vi "0 OCU.vi"(9 "Overview Image Ref In":T11, 10 "Map Name":T3="LPB Pool", 11 "Location of THINK":T14="127.0.0.1") -> ()   [LabVIEW 2011]
doc: "This is the current implementation of the operator control unit (OCU) for sailbot interfacing with this OCU over a network connection. The following features are currently implemented:\n- override control of the rudden angle and sail value by control interface or using keys\n- ability to add missions before and during a run, by clicking and by using GPS location of the boat or an auxiliary GPS attached to the OCU computer\n- modification of tuning values used on the boat\n- indicators for all relevant system status information\n\nAuthors: Jared Kirschner, Jason Curtis"
uses:
  2-Think/2 Typedefs/setpoints to boat.ctl
  2-Think/2 Typedefs/sail setpt.ctl
  2-Think/2 Typedefs/rudder angle.ctl
  2-Think/2 Typedefs/Velocity.ctl
  2-Think/2 Typedefs/apparent wind direction.ctl
  2-Think/2 Typedefs/apparent wind speed.ctl
  2-Think/2 Typedefs/apparent wind.ctl
  2-Think/2 Typedefs/heading.ctl
  2-Think/2 Typedefs/UTM Location.ctl
  2-Think/2 Typedefs/Which Boat.ctl
  2-Think/2 Typedefs/generalized sensor status.ctl
  2-Think/2 Typedefs/indicator LED.ctl
  0x2-OCU-Think Comm/0x2 Typedefs/Current Waypoint.ctl
  2-Think/2 Typedefs/robot velocity.ctl
  0x2-OCU-Think Comm/0x2 Typedefs/manual override.ctl
  0 Typedefs/Location of Think.ctl
  0 Typedefs/Sail Position.ctl
  0 Typedefs/Rudder Position.ctl
  0 Typedefs/Apparent Wind Point of Sail.ctl
  0x2-OCU-Think Comm/0x2 Typedefs/ocuWaypoint.ctl
  0x2-OCU-Think Comm/0x2 Typedefs/Waypoints List.ctl
  2-Think/2 Classes/Waypoint/Waypoint.lvclass
  0 Typedefs/Mission Type Radio Buttons.ctl
  2-Think/2 Typedefs/rate of turn.ctl
  2-Think/2 Typedefs/pitch and roll.ctl
  0 Typedefs/Maps.ctl
  <vilib>/vision/Image Controls.llb/IMAQ Image.ctl
  2-Think/2 Classes/Missions/GenericMission/GenericMission.lvclass
  2-Think/2 Typedefs/UTM Circle.ctl
  0x2-OCU-Think Comm/0x2 Typedefs/Control values.ctl
  2-Think/2 Typedefs/Goodness Weightings.ctl
  2-Think/2 Typedefs/PI Constants.ctl
  2-Think/2 Typedefs/Apparent Wind Mode.ctl
  0x2-OCU-Think Comm/0x2 Typedefs/Sail Setting Tuning.ctl
  2-Think/2 Typedefs/eStopCommand.ctl
  0x2-OCU-Think Comm/0x2 Typedefs/RIO-OCU update controls.ctl
  2-Think/2 Typedefs/generalized actuator status.ctl
  2-Think/2 Typedefs/absolute wind direction.ctl
  2-Think/2 Typedefs/absolute wind speed.ctl
  2-Think/2 Typedefs/absolute water current vector.ctl
  2-Think/2 Typedefs/Goodness Fns Indicator.ctl
  2-Think/2 Typedefs/tacking attempt.ctl
  0x2-OCU-Think Comm/0x2 Classes/NetworkStreams/Reader/readType.ctl
  0x2-OCU-Think Comm/0x2 Typedefs/ocuMessage.ctl
  0x2-OCU-Think Comm/0x2 Typedefs/ocuCommands.ctl
  2-Think/2 Globals/2 Global.vi
  0x2-OCU-Think Comm/OCUtoSim.vi
  0x2-OCU-Think Comm/0x2 Classes/NetworkStreams/Reader/NetworkStreamReader.lvclass
  0x2-OCU-Think Comm/0x2 Classes/NetworkStreams/Writer/NetworkStreamWriter.lvclass
  2-Think/2 Classes/Missions/RoundBuoy/RoundBuoy.lvclass
  2-Think/2 Classes/Missions/PassBuoys/PassBuoys.lvclass
  2-Think/2 Classes/Missions/StationKeeping/StationKeeping.lvclass
  2-Think/2 Classes/Missions/Drive/DriveTo.lvclass
panel:
  in  "Simulator controls":enum32{"Running", "Paused"}(tab)
  in  "Set Water Current Speed":dbl
  in  "Set Water Current Direction":dbl(knob) scale=0.0..360.0
  in  "Set Wind Speed":dbl=2.0
  in  "Pause Simulator?":bool
  in  "Set Wind Direction":dbl(knob) scale=0.0..360.0
  in  "Move boat?":bool
  in  "Set Boat Heading":dbl(knob) scale=0.0..360.0
  in  "Enable \nLocal GPS":bool
  out "Sensor Status":T1
  in  "GPS COM port":refnum<visa-resource-name>="COM1"
  in  "Additional inputs":T4(tab)
  in  "Manual Mission Input":enum32{"Drive", "Round", "Pass", "Station"}(tab)
  in  "Waypoint Location":enum32{"0", "1", "2", "3", "4"}(radio)
  in  "Buoy Side":enum32{"Starboard", "Port"}(radio)
  in  "Buoy to Round":enum32{"0", "1", "2", "3", "4"}(radio)
  in  "Starboard Buoy":enum32{"0", "1", "2", "3", "4"}(radio)=enum."1"
  in  "Port Buoy":enum32{"0", "1", "2", "3", "4"}(radio)
  in  "Buoy B":enum32{"0", "1", "2", "3", "4"}(radio)=enum."1"
  in  "Buoy A":enum32{"0", "1", "2", "3", "4"}(radio)
  in  "Add Mission":bool
  in  "Stored Locations Array":T5[](array[typedef])=[{"UTM Zone"=0.0, "Hemisphere"=enum."North", "East"=0.0, "North"=0.0}, {"UTM Zone"=0.0, "Hemisphere"=enum."North", "East"=0.0, "North"=0.0}, {"UTM Zone"=0.0, "Hemisphere"=enum."North", "East"=0.0, "North"=0.0}, {"UTM Zone"=0.0, "Hemisphere"=enum."North", "East"=0.0, "North"=0.0}, {"UTM Zone"=0.0, "Hemisphere"=enum."North", "East"=0.0, "North"=0.0}] {"North" format="%#_10f"; "East" format="%#_8f"}
  in  "Boat to Point 0":bool
  in  "Boat to Point 1":bool
  in  "Boat to Point 2":bool
  in  "Boat to Point 3":bool
  in  "Boat to Point 4":bool
  in  "Local to Point 4":bool
  in  "Local to Point 3":bool
  in  "Local to Point 2":bool
  in  "Local to Point 1":bool
  in  "Local to Point 0":bool
  in  "Update Constants":bool
  in  "Tuning Values":T6={"Goodness Weightings"={"Target Importance"=0.8, "No Sail Importance"=1.0, "Change Importance"=0.8, "Pure Waypoint \nImportance"=0.0, "Pure Wind \nImportance"=0.0}, "PI Constants"={"Proportional Gain"=0.5, "Integral Time"=0.0, "Derivative Time"=0.0}, "No Sail Zone\nTuning Quotient"=0.05, "Heading Change Wind Adjustment"=0.2, "Waypoint Tuning Quotient"=10.0, "Apparent Wind Mode"={"Desired Apparent\nWind Direction"=0.0, "On"=FALSE}, "Let Sail Out on Windcross"=TRUE, "Shift Goal for currents"=FALSE, "Round Buoy Safety"=5.0, "Sail Setting Options"={"Linear\nMode"=FALSE, "Sails Full In Point"=85.0, "Sails Full Out Point"=180.0}, "Defilter Wind Data"=TRUE, "Irons Range"=10.0, "Aggressiveness"=0.0} {"Aggressiveness" min=0.0 max=1.0; "Sail Setting Options"."Sails Full Out Point" step=0.1; "Sail Setting Options"."Sails Full In Point" step=0.1; "Apparent Wind Mode"."Desired Apparent\nWind Direction" step=0.1; "Goodness Weightings"."Pure Wind \nImportance" min=0.0 step=0.2; "Goodness Weightings"."Pure Waypoint \nImportance" min=0.0 step=0.2; "Goodness Weightings"."Change Importance" min=0.0 step=0.2; "Goodness Weightings"."No Sail Importance" min=0.0 step=0.2; "Goodness Weightings"."Target Importance" min=0.0 step=0.2}
  out "Battery Voltage":dbl
  out "Which Boat Am I?":T12
  out "Rudder Position":T13 scale=50.0..-50.0 scale format="%#.2g"
  out "Connected?":bool caption="Connection Status"
  in  "OVERRIDE SAIL?":bool
  in  "OVERRIDE RUDDER?":bool
  in  "Stop":bool
  in  "OCU Tab Control":enum32{"Mission [M]ap", "Detailed [T]elemetry"}(tab)
  in  "Map Mode":enum32{"M[i]ssion Edit", "M[o]nitoring"}(tab)
  in  "Load MDF":bool
  in  "Time(s)":dbl=300.0
  in  "Tolerance":dbl=3.0
  in  "Mission Entry Type":T15
  in  "Mission Def Filepath":path caption="MDF (Mission Definition File) path"
  in  "Reset Missions/Waypts":bool
  in  "Save Waypoints\nand PoI":bool
  out "Heading":T16 format="%05.1f"
  in  "Plot Colors":T17={"Target"=3381759, "No Sail"=16711680, "Change"=16756736, "Pure Waypt"=35080, "Pure Wind"=16860, "Combined"=16777228}
  out "Goodness Functions":picture
  out "Apparent Wind Direction\nPoint of Sail":T18 scale=0.0..360.0 scale format="%4d"
  out "Mission Status":string caption="Current Mission\nStatus"
  in  "Log message":string caption="Log message (type and press enter)"
  in  "Save Image":bool
  out "Mission Map":T11(plugin-control)
  in  "Overlay Font Size":i16=40
  out "# of Waypts":i32
  in  "Globals":T19(tab)
  out "Don't Tip?":bool
  out "Wind Sensor Status":T1
  out "Estimated Error":dbl
  out "Robot Heading":T16 format="%05.1f"
  out "Robot UTM Location":T5 {"North" format="%#_10f"; "East" format="%#_8f"}
  out "Robot Velocity":T20
  out "Robot\nRate of Turn":T21 format="%05.1f"
  out "Robot Pitch/Roll":T22 {"Roll" format="%05.1f"; "Pitch" format="%05.1f"}
  out "Robot Speed (m/s)":dbl
  out "Absolute Wind":T23 {"East" format="%#_5g"}
  out "Apparent Wind Direction":T24
  out "Apparent Wind Speed":T25
  out "Apparent Wind":T26
  out "Crossing Wind":bool
  out "Setpoints to boat":T27
  out "Sail Position":T28
  out "Rudder Angle":T29
  out "Current Waypoint":T30
  in  "Reset to start":bool
  out "Manual Override":T31
  out "Waypoints Array":T32[](array[typedef]) {"UTM Location"."North" format="%#_10f"; "UTM Location"."East" format="%#_8f"}
  out "Waypoints Object Array":T33
  out "Mission Object Array":refnum<class "GenericMission.lvclass">[](array[class])
  out "Global No Sail Circles":T34[](array[typedef])
  out "Sail Position":T35
  # "PORT"
  # "STARB"
  # "Local GPS"
  # "Note: if THINK\nis on this computer,\nturning on local GPS will do strange things."
  # "Note: the direction the current is coming from is opposite\n the dial. This is the direction the current is going to."
  # "When set,\nclick on map\nto move boat"
  # "HOWTO:\n1. save one or more points by moving GPS sensor to point, and pressing buttons below\n2. choose type of mission from tab control\n3. choose saved point(s) to load into mission. other params come from mission map input above\n4. click \"Add Mission\""
  # "P"
  # "S"
  # "O"
  # "O"
  # "A"
  # "B"
  # "HOWTO:\nchange values here, \nthen hit:"
  # "inputting missions:\nGo To Waypoint: set tolerance, and click on map.\nRound Buoy Port/Starboard: set tolerance, click.\nPass Between Buoys: Click one buoy location\nand drag to the other.\nStation Keeping: click southwest corner, drag to \nsoutheast corner. A square will be generated.\nTime(s) currently unimplemented.\nGlobal No-Sail Zone: click center of zone, drag to edge of\nzone. A circle with appropriate radius will be created."
  # "As Measured"
  # "Path Planning"
  # "From Planning Functions"
  # "(this is not a cluster because subitems\nare generated in parallel code)"
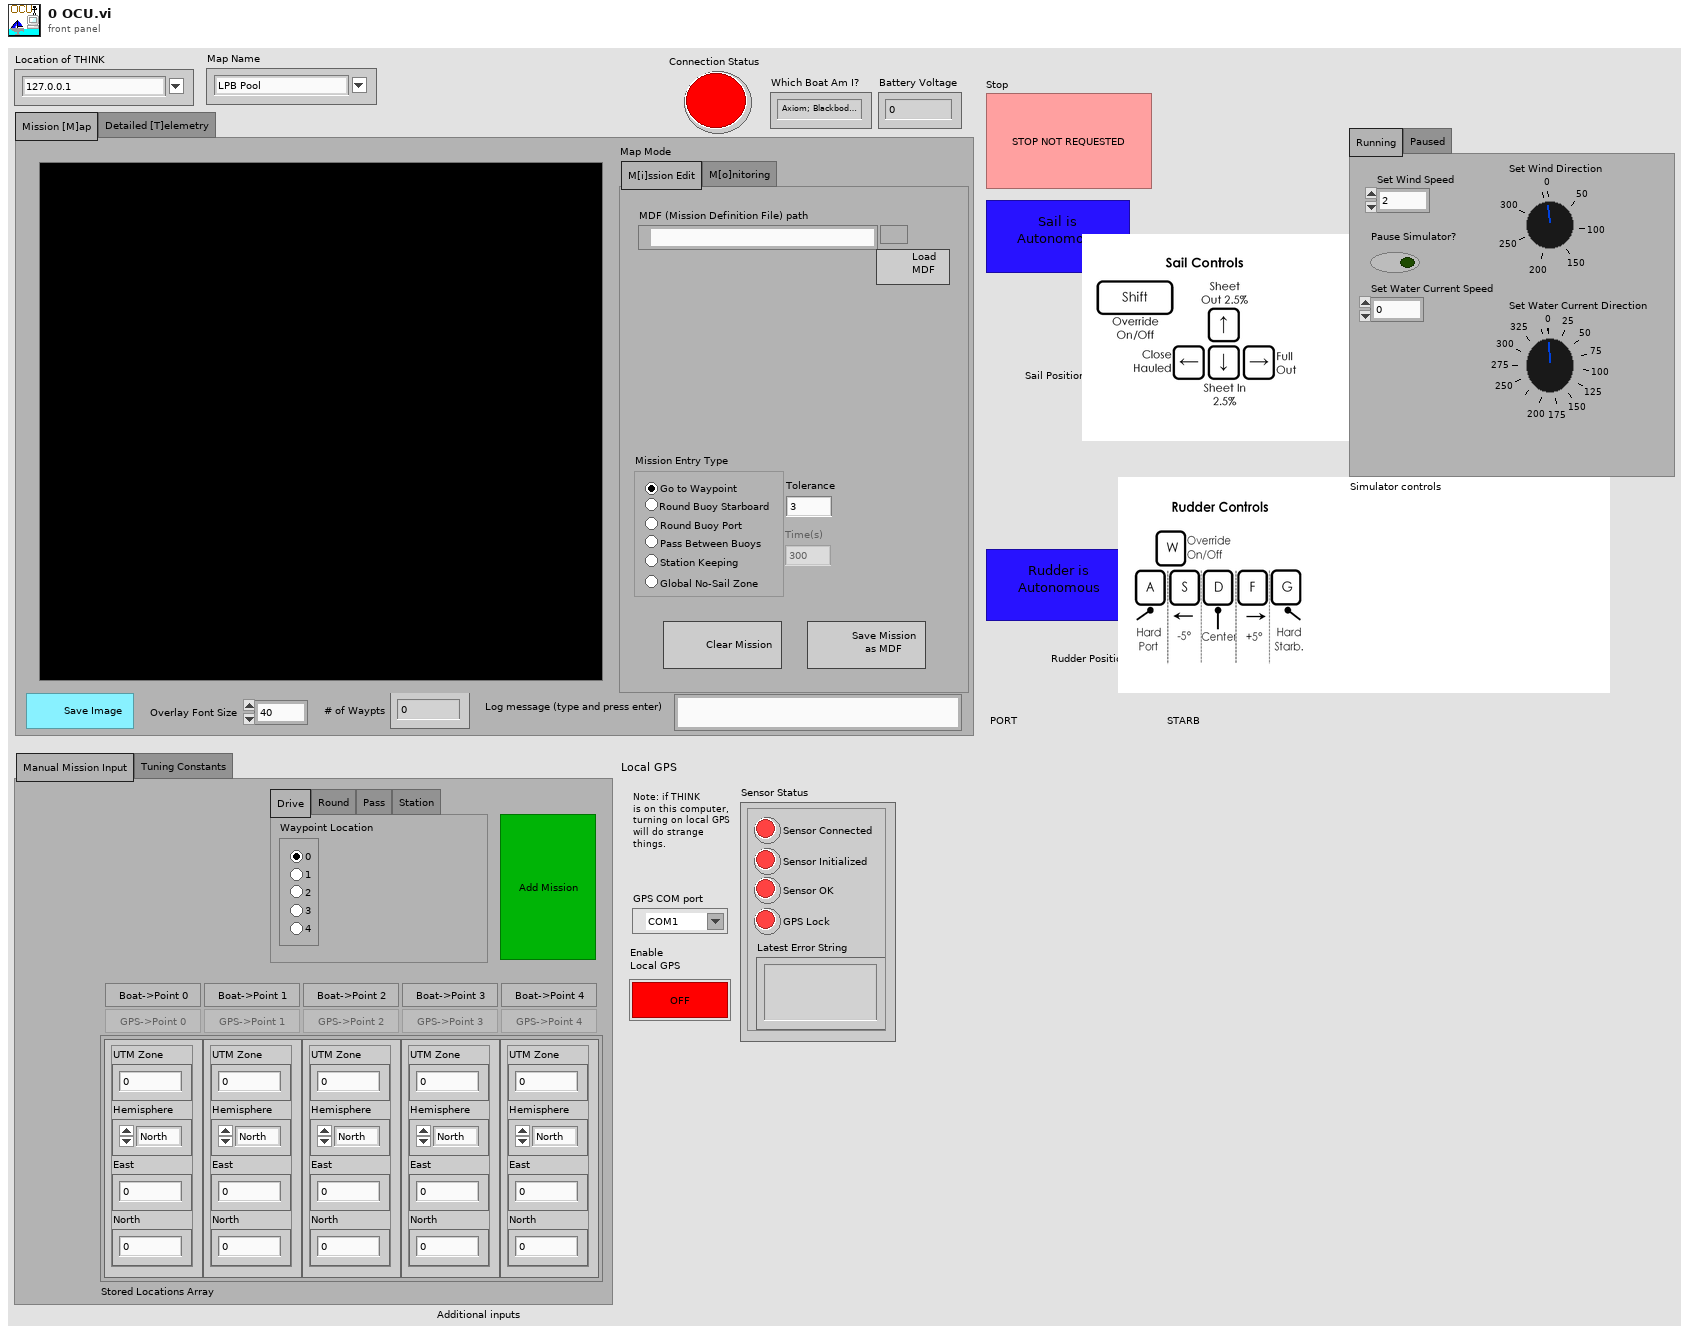
[diagram p1: front panel]
types:
  T1 = typedef "generalized sensor status.ctl" = cluster{"Sensor Connected":T2, "Sensor Initialized":T2, "Sensor OK":T2, "Latest Error String":string, "GPS Lock":T2}
  T2 = typedef "indicator LED.ctl" = bool
  T3 = typedef "Maps.ctl" = string
  T4 = enum32{"Manual Mission Input", "Tuning Constants"}
  T5 = typedef "UTM Location.ctl" = cluster{"UTM Zone":dbl, "Hemisphere":enum16{"North", "South"}, "East":dbl, "North":dbl}
  T6 = typedef "Control values.ctl" = cluster{"Goodness Weightings":T7, "PI Constants":T8, "No Sail Zone\nTuning Quotient":dbl, "Heading Change Wind Adjustment":dbl, "Waypoint Tuning Quotient":dbl, "Apparent Wind Mode":T9, "Let Sail Out on Windcross":bool, "Shift Goal for currents":bool, "Round Buoy Safety":dbl, "Sail Setting Options":T10, "Defilter Wind Data":bool, "Irons Range":dbl, "Aggressiveness":dbl}
  T7 = typedef "Goodness Weightings.ctl" = cluster{"Target Importance":dbl, "No Sail Importance":dbl, "Change Importance":dbl, "Pure Waypoint \nImportance":dbl, "Pure Wind \nImportance":dbl}
  T8 = typedef "PI Constants.ctl" = cluster{"Proportional Gain":dbl, "Integral Time":dbl, "Derivative Time":dbl}
  T9 = typedef "Apparent Wind Mode.ctl" = cluster{"Desired Apparent\nWind Direction":dbl, "On":bool}
  T10 = typedef "Sail Setting Tuning.ctl" = cluster{"Linear\nMode":bool, "Sails Full In Point":dbl, "Sails Full Out Point":dbl}
  T11 = typedef "IMAQ Image.ctl" = refnum<image>
  T12 = typedef "Which Boat.ctl" = enum16{"Axiom; Blackbody Radiation", "Simulation"}
  T13 = typedef "Rudder Position.ctl" = dbl
  T14 = typedef "Location of Think.ctl" = string
  T15 = typedef "Mission Type Radio Buttons.ctl" = enum32{"Go to Waypoint", "Round Buoy Starboard", "Round Buoy Port", "Pass Between Buoys", "Station Keeping", "Global No-Sail Zone"}
  T16 = typedef "heading.ctl" = dbl
  T17 = cluster{"Target":u32, "No Sail":u32, "Change":u32, "Pure Waypt":u32, "Pure Wind":u32, "Combined":u32}
  T18 = typedef "Apparent Wind Point of Sail.ctl" = dbl
  T19 = enum32{"How Am I", "Where Am I", "What's Around Me", "Path Planning"}
  T20 = typedef "robot velocity.ctl" = cluster{"East":dbl, "North":dbl}
  T21 = typedef "rate of turn.ctl" = dbl
  T22 = typedef "pitch and roll.ctl" = cluster{"Pitch":dbl, "Roll":dbl}
  T23 = typedef "Velocity.ctl" = cluster{"East":dbl, "North":dbl}
  T24 = typedef "apparent wind direction.ctl" = dbl
  T25 = typedef "apparent wind speed.ctl" = dbl
  T26 = typedef "apparent wind.ctl" = cluster{"Toward Fore":dbl, "Toward Starboard":dbl}
  T27 = typedef "setpoints to boat.ctl" = cluster{"Sail Position":T28, "Rudder Angle":T29}
  T28 = typedef "sail setpt.ctl" = dbl
  T29 = typedef "rudder angle.ctl" = dbl
  T30 = typedef "Current Waypoint.ctl" = i32
  T31 = typedef "manual override.ctl" = cluster{"Override Active Rudder":bool, "Setpoints":T27, "Override Active Sail":bool}
  T32 = typedef "ocuWaypoint.ctl" = cluster{"Tolerance (m)":dbl, "UTM Location":T5}
  T33 = typedef "Waypoints List.ctl" = refnum<class "Waypoint.lvclass">[]
  T34 = typedef "UTM Circle.ctl" = cluster{"UTM Zone":dbl, "Hemisphere":enum16{"North", "South"}, "East":dbl, "North":dbl, "Radius":dbl}
  T35 = typedef "Sail Position.ctl" = dbl
  T36 = typedef "RIO-OCU update controls.ctl" = cluster{"Sensor Status":T1, "Battery Voltage":dbl, "Rudder Actuator Status":T37, "Sail Actuator Status":T37, "Which Boat Am I?":T12, "Robot Velocity":T20, "Robot UTM Location":T5, "Robot\nHeading ":T16, "Robot\nRate of Turn":T21, "Robot Pitch/Roll":T22, "Apparent Wind":T26, "Apparent Wind\nSpeed":T25, "Apparent Wind\nDirection (º)":T24, "Absolute Wind":T23, "Absolute Wind\nDirection (º)":T38, "Absolute Wind\nSpeed":T39, "Absolute Water Current Vector":T40, "Rudder Angle":T29, "Sail Position":T28, "Manual Override Cluster":T31, "Setpoints to boat":T27, "Current Waypoint":T30, "Think freq.":dbl, "Sense freq.":dbl, "Act freq.":dbl, "E-stop freq.":dbl, "Network \nfreq.":dbl, "Network \nLoop Iterations":i64, "E-Stop":bool, "Serialized Waypoint Array":string, "Serialized Mission Queue Elements":string, "Goodness Functions":T41, "Global No Sail Circles":T34[], "Optimal Heading":dbl, "Crossing Wind":bool, "Estimated Error":dbl, "Don't Tip?":bool, "Tacking Attempt":T42}
  T37 = typedef "generalized actuator status.ctl" = cluster{"Actuator Connected":T2}
  T38 = typedef "absolute wind direction.ctl" = dbl
  T39 = typedef "absolute wind speed.ctl" = dbl
  T40 = typedef "absolute water current vector.ctl" = cluster{"Direction":T24, "Magnitude":T24}
  T41 = typedef "Goodness Fns Indicator.ctl" = cluster{dbl, dbl, dbl[][]}
  T42 = typedef "tacking attempt.ctl" = cluster{"attempting tack":bool, "tacking attempt\ntime remaining":dbl}
  T43 = typedef "0-Image Descriptor.ctl" = cluster{"Upper-Left Corner Coordinates":T5, "Meters/Pixel":dbl}
  T44 = typedef "eStopCommand.ctl" = enum16{"Reset E-Stop", "Get E-Stop", "Set E-Stop"}
  T45 = typedef "ocuMessage.ctl" = cluster{"OCU Command":T46, "Data":variant}
  T46 = typedef "ocuCommands.ctl" = enum16{"Pass", "Send override", "Set waypoint number", "Stop", "Add Mission", "Reset Missions/Waypts", "Edit Control Values", "Add Global No-Sail", "Log Message"}
  T47 = enum8{"Enabled", "Disabled", "Disabled and Grayed Out"}
  T48 = typedef "eventvkey.ctl" = enum16{"ASCII", "Enter", "Return", "Shift", "Ctrl", "Alt", "Cmd", "Opt", "Caps", "NumLock", "Clear", "Break", "Up", "Down", "Left", "Right", "Insert", "Delete", "Home", "End", "PageUp", "PageDown", "Escape", "Help", "Pause", "ScrollLock", "F1", "F2", "F3", "F4", "F5", "F6", "F7", "F8", "F9", "F10", "F11", "F12", "F13", "F14", "F15", "F16", "F17", "F18", "F19", "F20", "F21", "F22", "F23", "F24", "Play", "VolumeUp", "VolumeDown", "Mute", "Two Byte Char"}
  T49 = cluster{"Global Rectangle":i32[], "Contours":cluster{"Contour Type":u32, "ROI Type":u32, "Points":i32[]}[]}
  T50 = typedef "NetworkStreamReader.lvclass/readType.ctl" = enum16{"Next in buffer", "Most current"}
  T51 = cluster{"Image Ref Out":T11, "Image Descriptor":T43}
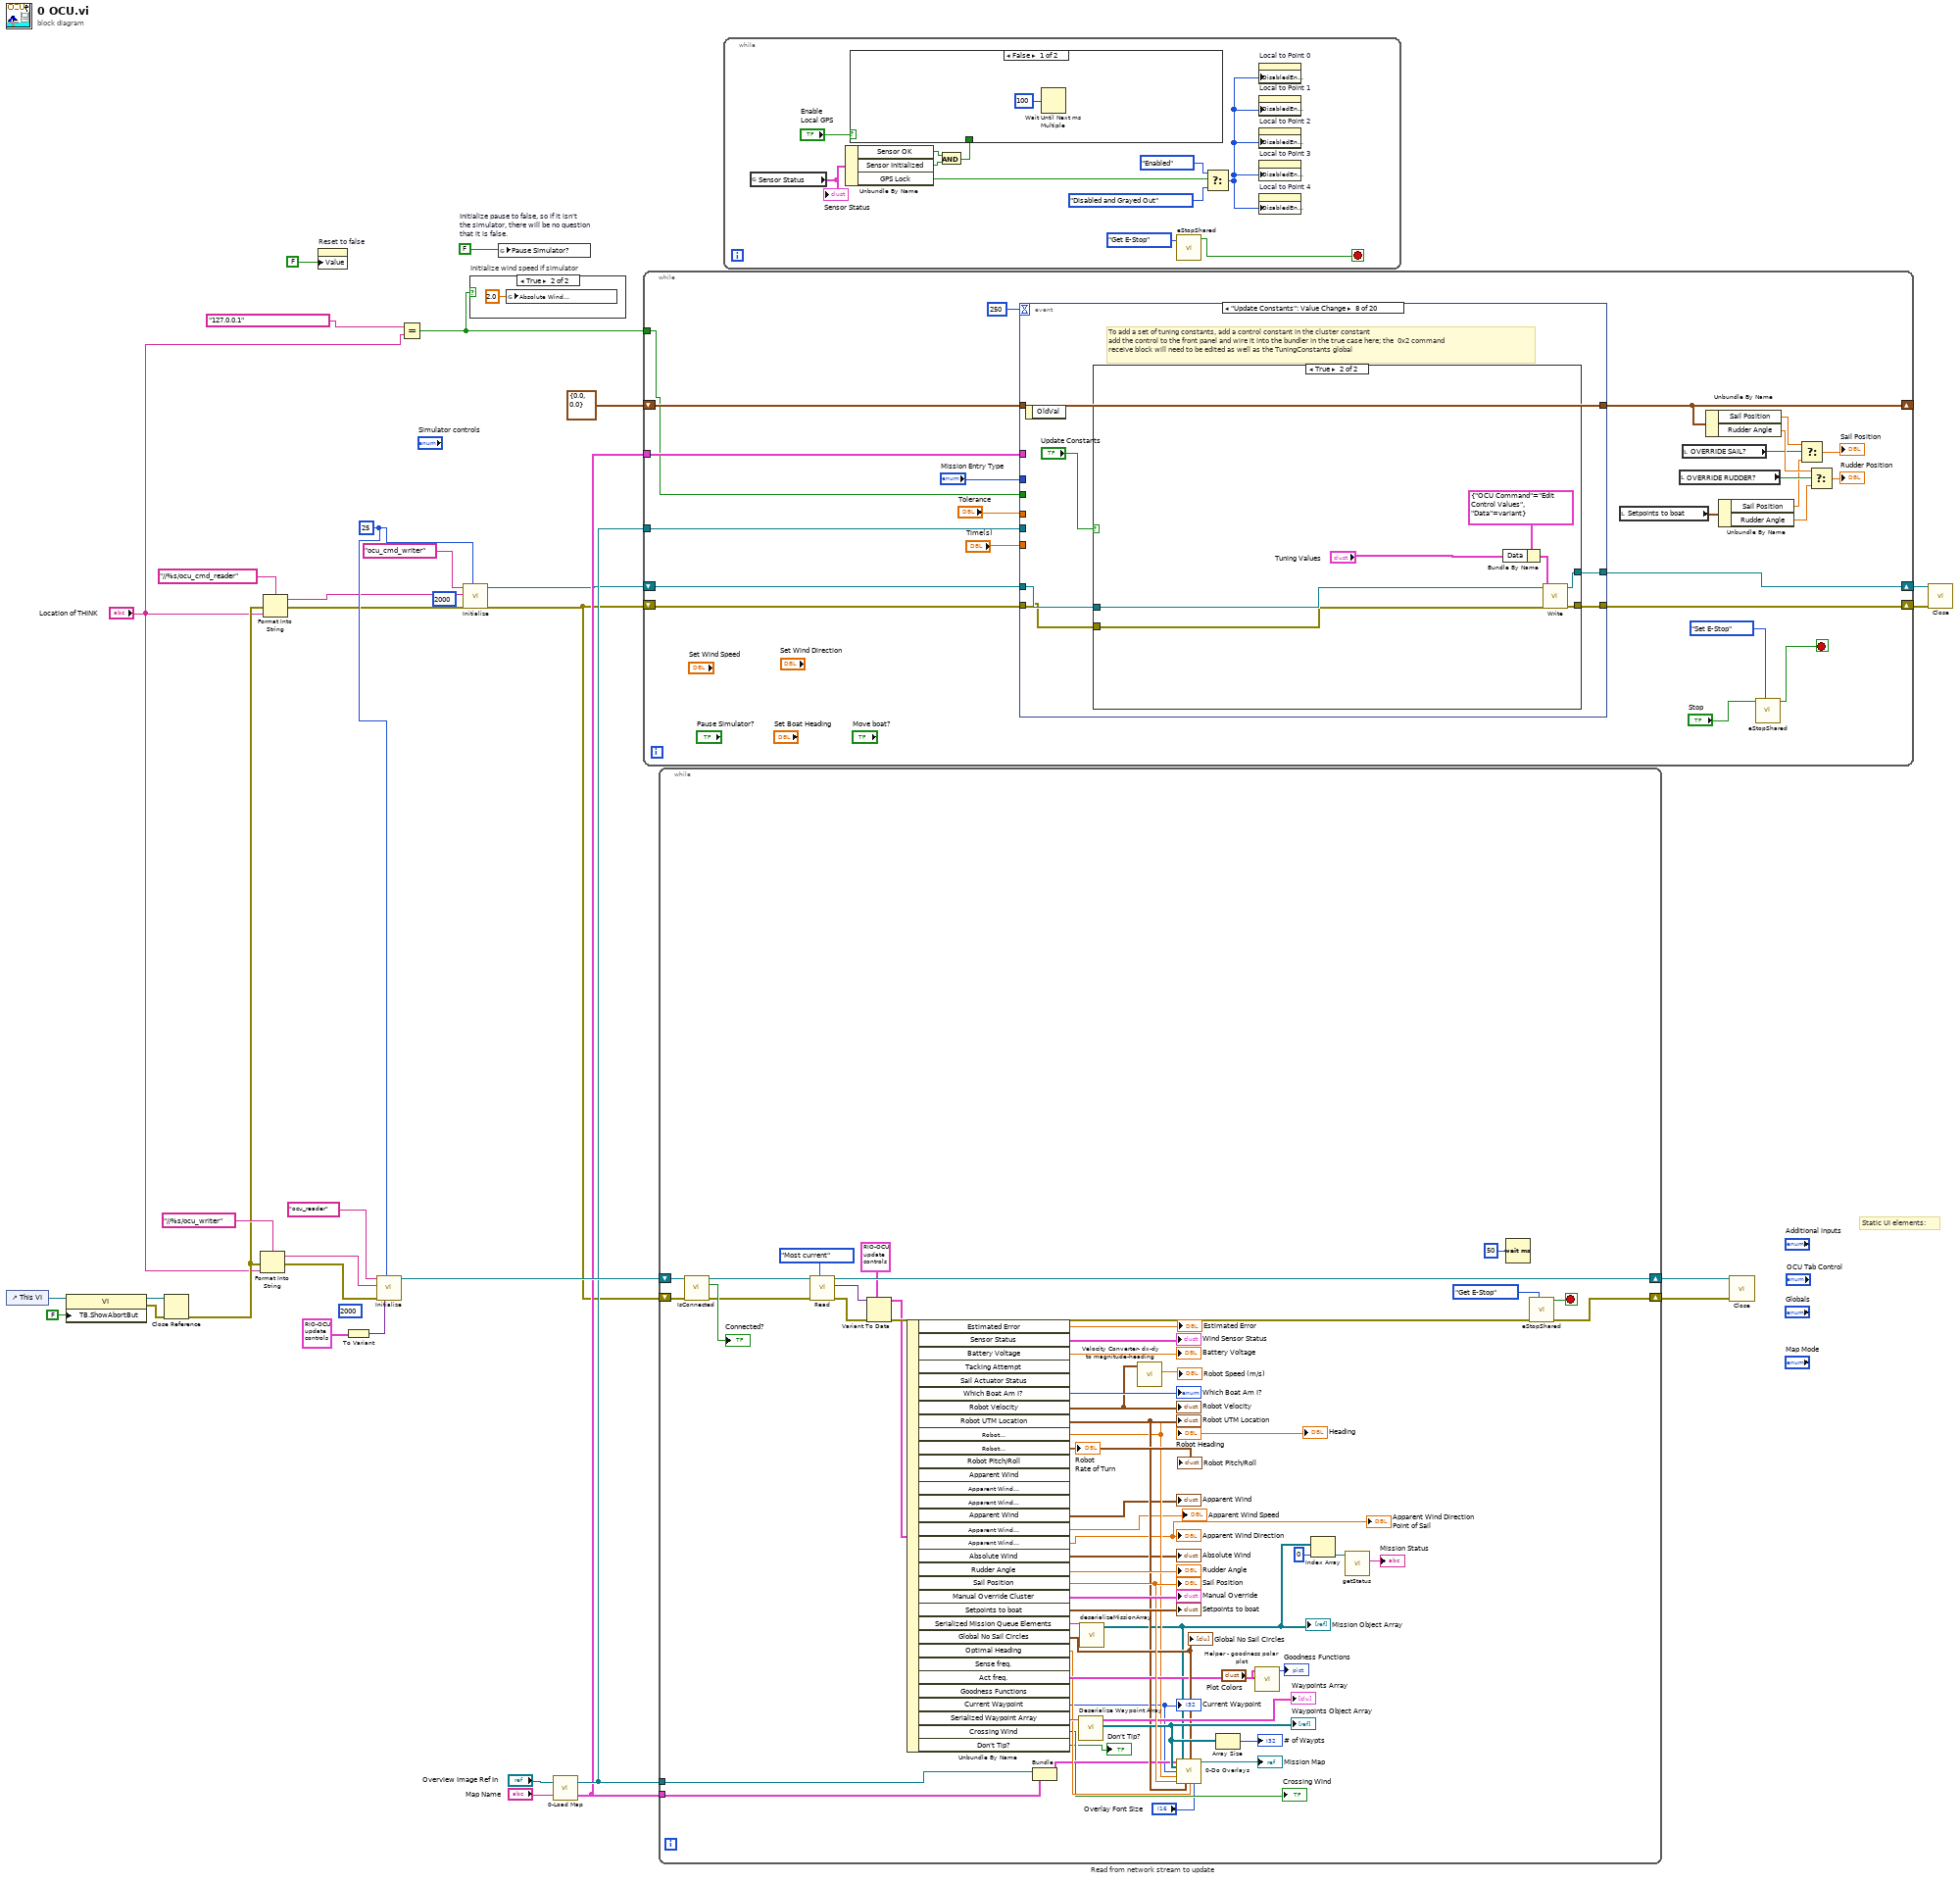
[diagram p0: block diagram]
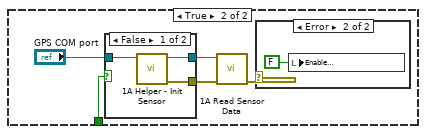
[diagram p3: hidden frame]
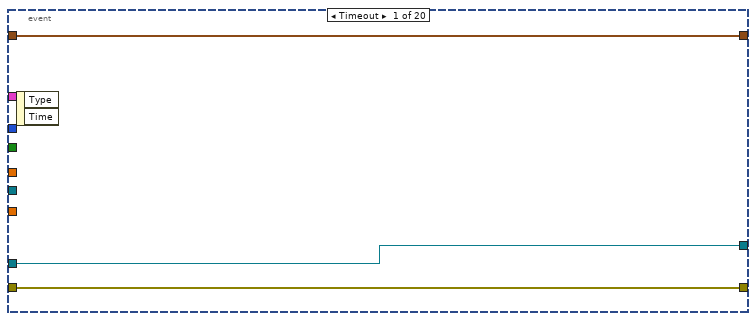
[diagram p6: hidden frame]
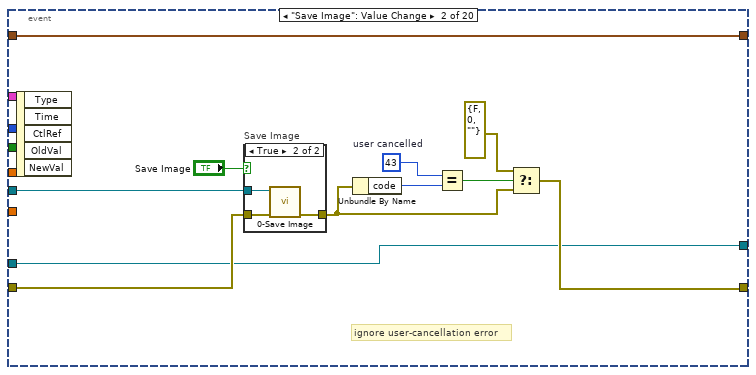
[diagram p7: hidden frame]
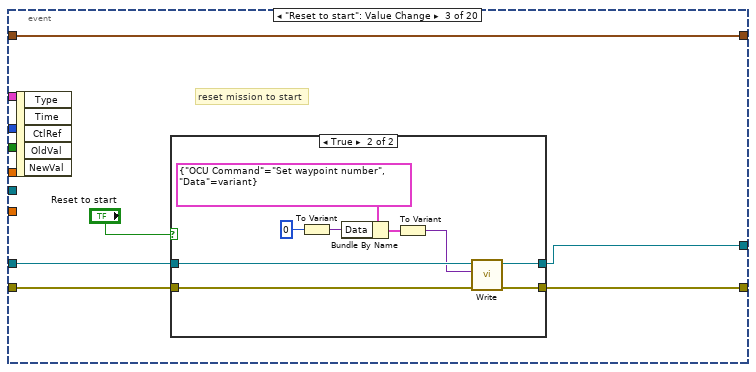
[diagram p9: hidden frame]
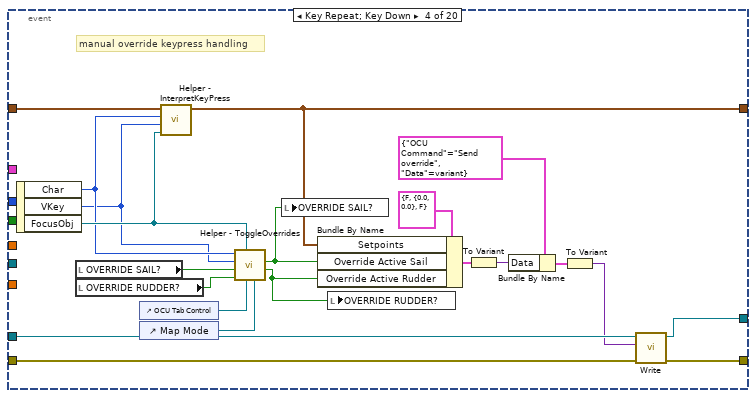
[diagram p11: hidden frame]
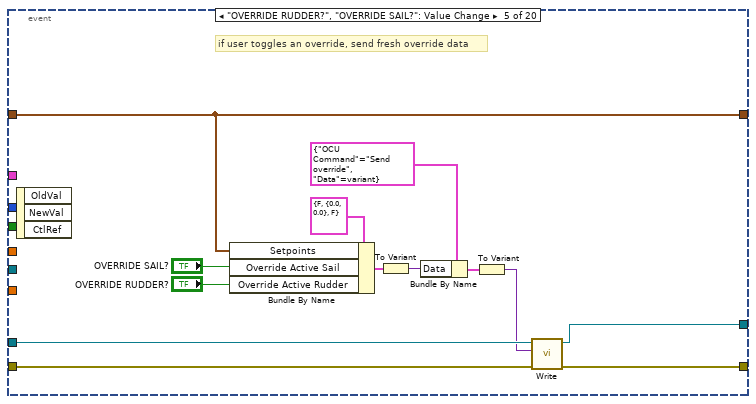
[diagram p12: hidden frame]
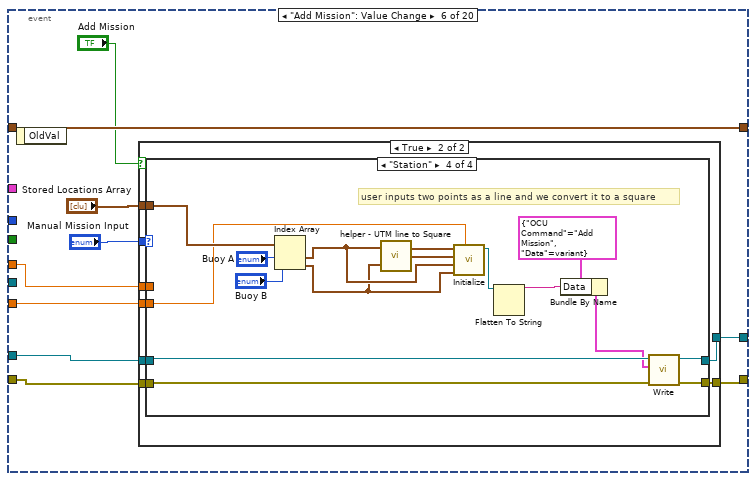
[diagram p13: hidden frame]
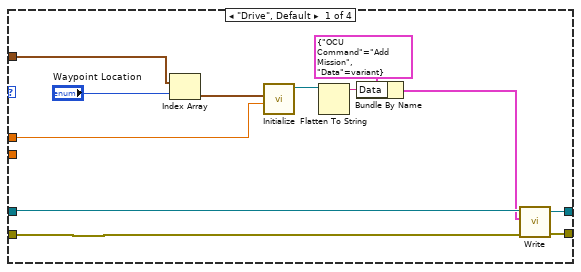
[diagram p15: hidden frame]
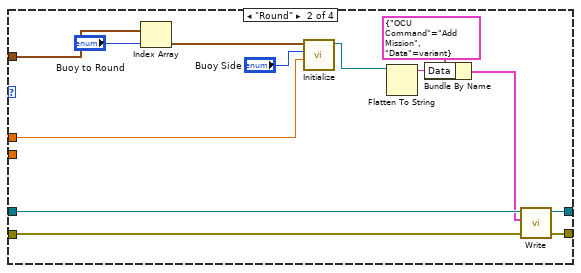
[diagram p16: hidden frame]
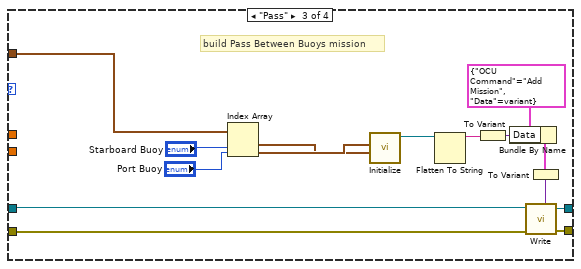
[diagram p17: hidden frame]
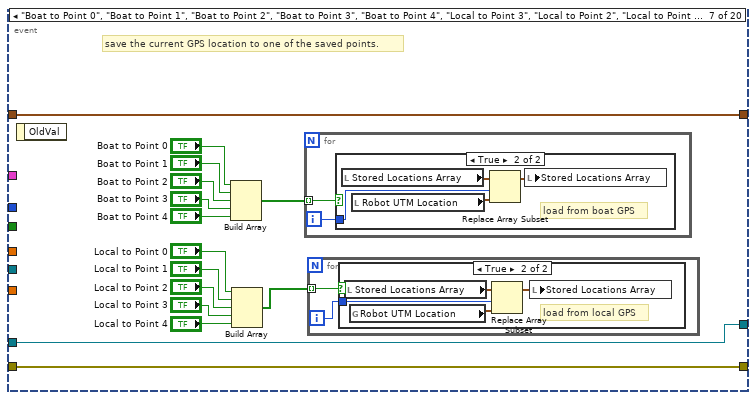
[diagram p18: hidden frame]
diagram:
  w3 = FALSE  # Initialize pause to false, so if it isn't the simulator, there will be no question that it is false.
  (unwired) 2000 ("connection timeout")
  (unwired) 2000 ("connection timeout")
  w31 = 25 ("writer buffer size")
  # "Static UI elements:"
  n1 = control-ref of="This VI"() -> (w22:refnum<vi>)
  n2 = property class="VI"(reference=w22, "TB.ShowAbortBut"=FALSE ("Tool Bar:Show Abort Button")) -> (reference out=w20:refnum<vi>, error out=w19:errorcluster)  [unwired: 1 in]
  n3 = Close Reference(reference=w20, error in (no error)=w19) -> (error out=w18:errorcluster)
  n4 = Format Into String(format string="//%s/ocu_writer", error in=w18, "Location of THINK") -> (resulting string=w12:string, error out=w16:errorcluster)  [unwired: 1 in]
  n5 = Format Into String(format string="//%s/ocu_cmd_reader", error in=w18, "Location of THINK") -> (resulting string=w10:string, error out=w17:errorcluster)  [unwired: 1 in]
  n6 = property on="Reset to false" class="Bool (strict)"("Value"=FALSE ("Pause Simulator?")) -> ()  [unwired: 2 in, 2 out]
  n7 = To Variant(anything=T36 {"Sensor Status"={"Sensor Connected"=FALSE, "Sensor Initialized"=FALSE, "Sensor OK"=FALSE, "Latest Error String"="", "GPS Lock"=FALSE}, "Battery Voltage"=0.0, "Rudder Actuator Status"={"Actuator Connected"=FALSE}, "Sail Actuator Status"={"Actuator Connected"=FALSE}, "Which Boat Am I?"=enum."Axiom; Blackbody Radiation", "Robot Velocity"={"East"=0.0, "North"=0.0}, "Robot UTM Location"={"UTM Zone"=0.0, "Hemisphere"=enum."North", "East"=0.0, "North"=0.0}, "Robot\nHeading "=0.0, "Robot\nRate of Turn"=0.0, "Robot Pitch/Roll"={"Pitch"=0.0, "Roll"=0.0}, "Apparent Wind"={"Toward Fore"=0.0, "Toward Starboard"=0.0}, "Apparent Wind\nSpeed"=0.0, "Apparent Wind\nDirection (º)"=0.0, "Absolute Wind"={"East"=0.0, "North"=0.0}, "Absolute Wind\nDirection (º)"=0.0, "Absolute Wind\nSpeed"=0.0, "Absolute Water Current Vector"={"Direction"=0.0, "Magnitude"=0.0}, "Rudder Angle"=0.0, "Sail Position"=0.0, "Manual Override Cluster"={"Override Active Rudder"=FALSE, "Setpoints"={"Sail Position"=0.0, "Rudder Angle"=0.0}, "Override Active Sail"=FALSE}, "Setpoints to boat"={"Sail Position"=0.0, "Rudder Angle"=0.0}, "Current Waypoint"=0, "Think freq."=0.0, "Sense freq."=0.0, "Act freq."=0.0, "E-stop freq."=0.0, "Network \nfreq."=0.0, "Network \nLoop Iterations"=0, "E-Stop"=FALSE, "Serialized Waypoint Array"="", "Serialized Mission Queue Elements"="", "Goodness Functions"={0.0, 0.0, []}, "Global No Sail Circles"=[], "Optimal Heading"=0.0, "Crossing Wind"=FALSE, "Estimated Error"=0.0, "Don't Tip?"=FALSE, "Tacking Attempt"={"attempting tack"=FALSE, "tacking attempt\ntime remaining"=0.0}} ("RIO->OCU update data")) -> (Variant=w30:variant)
  n8 = call "Initialize.vi"("Default return"=w30, "reader buffer size"=w31, "error in (no error)"=w16, "writer url"=w12, "reader name"="ocu_reader" ("writer name")) -> ("NetworkStreamWriter out"=w32:refnum<class "NetworkStreamReader.lvclass">)  [unwired: 5 in, 1 out]
  n9 = Equal?(x=T14 "127.0.0.1" ("y"), y="Location of THINK") -> (x = y?=w2:bool)
  n10 = call "Initialize.vi"("writer buffer size"=w31, "error in (no error)"=w17, "reader url"=w10, "writer name"="ocu_cmd_writer") -> ("error out"=w6:errorcluster, "NetworkStreamWriter out"=w7:refnum<class "NetworkStreamWriter.lvclass">)  [unwired: 6 in]
  n11 = case "Initialize wind speed if simulator" shown="True" w2 {
    frame False {
    }
    frame True {
      n12 = global write "2 Global.vi" "Absolute Wind\nSpeed"(T39 2.0 ("Absolute Wind\nSpeed")) -> ()
    }
  }
  n13 = global write "OCUtoSim.vi" "Pause Simulator?"(w3) -> ()
  n14 = call "0-Load Map.vi"("Map Name"="Map Name", "Image Ref In"="Overview Image Ref In") -> ("Image Descriptor"=w14:T43, "Image Ref Out"=w27:T11)
  n15 = while {
    shift-right: [w58] -> w23
    shift-left: w6 -> [w40]
    shift-right: [w52] -> _
    shift-left: T27 {"Sail Position"=0.0, "Rudder Angle"=0.0} ("Setpoints") -> [w59]
    shift-right: [w54] -> w24
    shift-left: w7 -> [w41]
    tunnel: w27 -> [w53]
    tunnel: w14 -> [w51]
    tunnel: w2 -> [w35]
    stop <- w57 stop-if-true
    n16 = event shown="[7] \"Update Constants\": Value Change" {
      selector: _ -> [_ _ _ _ _ _ _ _ _ _ _ _ _ _ _ _ _ _ _ _]
      dyn-events: _ -> [_ _ _ _ _ _ _ _ _ _ _ _ _ _ _ _ _ _ _ _]
      timeout: 250 -> [_ _ _ _ _ _ _ _ _ _ _ _ _ _ _ _ _ _ _ _]
      tunnel: w59 -> [w62 w69 w83 w115 w118 w136 w212 w236 w258 w274 w283 w324 w334 w358 w504 w511 w520 w530 w542 w547]
      tunnel: [w62 w69 w83 w113 w118 w136 w212 w236 w258 w274 w283 w324 w334 w358 w504 w511 w520 w530 w542 w547] -> w52
      tunnel: w40 -> [w60 w67 w80 w110 w125 w137 w210 w233 w250 w273 w281 w322 w335 w357 w502 w509 w518 w528 w540 w549]
      tunnel: [w60 w64 w78 w109 w124 w134 w210 w231 w248 w273 w280 w320 w335 w355 w502 w509 w518 w528 w540 w549] -> w58
      tunnel: w41 -> [w61 w63 w81 w112 w127 w138 w211 w234 w249 w272 w279 w323 w336 w353 w503 w510 w519 w529 w541 w548]
      tunnel: [w61 w63 w79 w111 w126 w133 w211 w232 w251 w272 w278 w321 w336 w354 w503 w510 w519 w529 w541 w548] -> w54
      tunnel: w53 -> [_ w68 _ _ _ _ _ _ _ _ _ _ _ _ _ _ _ _ _ _]
      tunnel: w51 -> [_ _ _ _ _ _ _ _ _ _ _ _ _ w356 _ _ _ _ _ _]
      tunnel: "Mission Entry Type" -> [_ _ _ _ _ _ _ _ _ _ _ _ _ w352 _ _ _ _ _ _]
      tunnel: "Tolerance" -> [_ _ _ _ _ w135 _ _ _ _ _ _ _ w351 _ _ _ _ _ _]
      tunnel: "Time(s)" -> [_ _ _ _ _ w129 _ _ _ _ _ _ _ w350 _ _ _ _ _ _]
      tunnel: w35 -> [_ _ _ _ _ _ _ _ _ _ _ _ _ _ w500 w514 w524 w527 w544 w554]
      event Timeout {
        n17 = event-data() -> ()  [unwired: 1 in, 2 out]
      }
      event "Save Image": Value Change {
        w72 = 43  # user cancelled
        # "ignore user-cancellation error"
        n18 = event-data() -> ()  [unwired: 1 in, 5 out]
        n19 = case "Save Image" shown="True" "Save Image" {
          tunnel: w67 -> [w74 w77]
          tunnel: [w74 w76] -> w66
          tunnel: w68 -> [_ w75]
          frame False {
          }
          frame True {
            n20 = call "0-Save Image.vi"("Error In"=w77, "Image in"=w75) -> ("Error Out"=w76:errorcluster)  [unwired: 9 in]
          }
        }
        n21 = Unbundle By Name(w66) -> ("code"=w73:i32)
        n22 = Equal?(x=w72, y=w73) -> (x = y?=w71:bool)
        n23 = Select(t=errorcluster {"status"=FALSE, "code"=0, "source"=""}, s=w71, f=w66) -> (s? t:f=w64:errorcluster)
      }
      event "Reset to start": Value Change {
        # "reset mission to start"
        n24 = event-data() -> ()  [unwired: 1 in, 5 out]
        n25 = case shown="True" "Reset to start" {
          tunnel: w81 -> [w85 w91]
          tunnel: w80 -> [w84 w92]
          tunnel: [w85 w94] -> w79
          tunnel: [w84 w93] -> w78
          frame False {
          }
          frame True {
            n26 = To Variant(anything=T30 0 ("Current Waypoint")) -> (Variant=w89:variant)
            n27 = Bundle By Name(cluster=T45 {"OCU Command"=enum."Set waypoint number", "Data"=variant}, "Data"=w89) -> (w87:T45)
            n28 = To Variant(anything=w87) -> (Variant=w86:variant)
            n29 = call "Write.vi"("error in (no error)"=w92, "element"=w86, "NetworkStreamWriter in"=w91) -> ("error out"=w93:errorcluster, "NetworkStreamWriter out"=w94:refnum<class "NetworkStreamWriter.lvclass">)  [unwired: 7 in]
          }
        }
      }
      event Key Repeat; Key Down {
        # "manual override keypress handling"
        n30 = event-data() -> ("Char"=w102:i16, "VKey"=w101:T48, "FocusObj"=w103:refnum<vi>)  [unwired: 1 in]
        n31 = local read "OVERRIDE SAIL?"() -> (w100:bool)
        n32 = local read "OVERRIDE RUDDER?"() -> (w99:bool)
        n33 = control-ref of="OCU Tab Control"() -> (w96:refnum<vi>)
        n34 = control-ref of="Map Mode"() -> (w95:refnum<vi>)
        n35 = call "Helper - InterpretKeyPress.vi"("FocusObj"=w103, "VKey"=w101, "Char"=w102, "Command In"=w115) -> ("Command Out"=w113:T27)  [unwired: 7 in]
        n36 = call "Helper - ToggleOverrides.vi"("Map Mode Tab Control Ref"=w95, "OCU Tab Control Ref"=w96, "FocusObj"=w103, "Rudder Override?"=w99, "Sail Override?"=w100, "VKey"=w101, "Char"=w102) -> ("Override Rudder"=w98:bool, "Override Sail"=w97:bool)  [unwired: 3 in]
        n37 = local write "OVERRIDE SAIL?"(w97) -> ()
        n38 = Bundle By Name(cluster=T31 {"Override Active Rudder"=FALSE, "Setpoints"={"Sail Position"=0.0, "Rudder Angle"=0.0}, "Override Active Sail"=FALSE} ("Manual Override Cluster"), "Setpoints"=w113, "Override Active Sail"=w97, "Override Active Rudder"=w98) -> (w105:T31)
        n39 = local write "OVERRIDE RUDDER?"(w98) -> ()
        n40 = To Variant(anything=w105) -> (Variant=w108:variant)
        n41 = Bundle By Name(cluster=T45 {"OCU Command"=enum."Send override", "Data"=variant}, "Data"=w108) -> (w107:T45)
        n42 = To Variant(anything=w107) -> (Variant=w104:variant)
        n43 = call "Write.vi"("error in (no error)"=w110, "element"=w104, "NetworkStreamWriter in"=w112) -> ("error out"=w109:errorcluster, "NetworkStreamWriter out"=w111:refnum<class "NetworkStreamWriter.lvclass">)  [unwired: 7 in]
      }
      event "OVERRIDE RUDDER?", "OVERRIDE SAIL?": Value Change {
        # "if user toggles an override, send fresh override data"
        n44 = event-data() -> ()  [unwired: 1 in, 3 out]
        n45 = Bundle By Name(cluster=T31 {"Override Active Rudder"=FALSE, "Setpoints"={"Sail Position"=0.0, "Rudder Angle"=0.0}, "Override Active Sail"=FALSE} ("Manual Override Cluster"), "Setpoints"=w118, "Override Active Sail"="OVERRIDE SAIL?", "Override Active Rudder"="OVERRIDE RUDDER?") -> (w120:T31)
        n46 = To Variant(anything=w120) -> (Variant=w123:variant)
        n47 = Bundle By Name(cluster=T45 {"OCU Command"=enum."Send override", "Data"=variant}, "Data"=w123) -> (w122:T45)
        n48 = To Variant(anything=w122) -> (Variant=w119:variant)
        n49 = call "Write.vi"("error in (no error)"=w125, "element"=w119, "NetworkStreamWriter in"=w127) -> ("error out"=w124:errorcluster, "NetworkStreamWriter out"=w126:refnum<class "NetworkStreamWriter.lvclass">)  [unwired: 7 in]
      }
      event "Add Mission": Value Change {
        n50 = event-data() -> ()  [unwired: 1 in, 1 out]
        n51 = case shown="True" "Add Mission" {
          tunnel: w138 -> [w140 w148]
          tunnel: w137 -> [w139 w147]
          tunnel: w135 -> [_ w146]
          tunnel: [w139 w145] -> w134
          tunnel: [w140 w144] -> w133
          tunnel: "Manual Mission Input" -> [_ w143]
          tunnel: "Stored Locations Array" -> [_ w142]
          tunnel: w129 -> [_ w141]
          frame False {
          }
          frame True {
            n52 = case shown="\"Station\"" w143 {
              tunnel: w147 -> [w156 w169 w178 w196]
              tunnel: [w160 w169 w181 w201] -> w145
              tunnel: w146 -> [w157 w172 _ _]
              tunnel: [w159 w171 w182 w202] -> w144
              tunnel: w148 -> [w158 w170 w183 w200]
              tunnel: w142 -> [w151 w167 w177 w195]
              tunnel: w141 -> [_ _ _ w188]
              frame "Drive", Default {
                n53 = Index Array(array=w151, index="Waypoint Location") -> (element=w154:T5)
                n54 = call "Initialize.vi"("Tolerance (m)"=w157, "Drive Location"=w154) -> ("Drive out"=w152:refnum<class "DriveTo.lvclass">)  [unwired: 8 in, 1 out]
                n55 = Flatten To String(anything=w152) -> (data string=w150:string)  [unwired: 3 in, 2 out]
                n56 = Bundle By Name(cluster=T45 {"OCU Command"=enum."Add Mission", "Data"=variant}, "Data"=w150) -> (w149:T45)
                n57 = call "Write.vi"("error in (no error)"=w156, "element"=w149, "NetworkStreamWriter in"=w158) -> ("error out"=w160:errorcluster, "NetworkStreamWriter out"=w159:refnum<class "NetworkStreamWriter.lvclass">)  [unwired: 7 in]
              }
              frame "Round" {
                n58 = Index Array(array=w167, index="Buoy to Round") -> (element=w166:T5)
                n59 = call "Initialize.vi"("Tolerance (m)"=w172, "Round side?"="Buoy Side", "Buoy to Round"=w166) -> ("RoundBuoys out"=w161:refnum<class "RoundBuoy.lvclass">)  [unwired: 7 in, 1 out]
                n60 = Flatten To String(anything=w161) -> (data string=w163:string)  [unwired: 3 in, 2 out]
                n61 = Bundle By Name(cluster=T45 {"OCU Command"=enum."Add Mission", "Data"=variant}, "Data"=w163) -> (w162:T45)
                n62 = call "Write.vi"("element"=w162, "NetworkStreamWriter in"=w170) -> ("NetworkStreamWriter out"=w171:refnum<class "NetworkStreamWriter.lvclass">)  [unwired: 8 in, 1 out]
              }
              frame "Pass" {
                # "build Pass Between Buoys mission"
                n63 = Index Array(array=w177, index #1="Starboard Buoy", index #2="Port Buoy") -> (element #1=w173:T5, element #2=w174:T5)
                n64 = call "Initialize.vi"("Buoy Pass 2"=w173, "Buoy Pass 1"=w174) -> ("PassBuoys out"=w179:refnum<class "PassBuoys.lvclass">)  [unwired: 8 in, 1 out]
                n65 = Flatten To String(anything=w179) -> (data string=w185:string)  [unwired: 3 in, 2 out]
                n66 = To Variant(anything=w185) -> (Variant=w186:variant)
                n67 = Bundle By Name(cluster=T45 {"OCU Command"=enum."Add Mission", "Data"=variant}, "Data"=w186) -> (w184:T45)
                n68 = To Variant(anything=w184) -> (Variant=w180:variant)
                n69 = call "Write.vi"("error in (no error)"=w178, "element"=w180, "NetworkStreamWriter in"=w183) -> ("error out"=w181:errorcluster, "NetworkStreamWriter out"=w182:refnum<class "NetworkStreamWriter.lvclass">)  [unwired: 7 in]
              }
              frame "Station" {
                # "user inputs two points as a line and we convert it to a square"
                n70 = Index Array(array=w195, index #1="Buoy A", index #2="Buoy B") -> (element #1=w192:T5, element #2=w191:T5)
                n71 = call "helper - UTM line to Square.vi"("Endpoint 2, UTM"=w191, "Endpoint 1, UTM"=w192) -> ("Endpoint 4, UTM"=w198:T5, "Endpoint 3, UTM"=w197:T5)
                n72 = call "Initialize.vi"("Duration (s)"=w188, "Buoy SE"=w191, "Buoy SW"=w192, "Buoy NE"=w198, "Buoy NW"=w197) -> ("StationKeeping out"=w199:refnum<class "StationKeeping.lvclass">)  [unwired: 5 in, 1 out]
                n73 = Flatten To String(anything=w199) -> (data string=w190:string)  [unwired: 3 in, 2 out]
                n74 = Bundle By Name(cluster=T45 {"OCU Command"=enum."Add Mission", "Data"=variant}, "Data"=w190) -> (w189:T45)
                n75 = call "Write.vi"("error in (no error)"=w196, "element"=w189, "NetworkStreamWriter in"=w200) -> ("error out"=w201:errorcluster, "NetworkStreamWriter out"=w202:refnum<class "NetworkStreamWriter.lvclass">)  [unwired: 7 in]
              }
            }
          }
        }
      }
      event "Boat to Point 0", "Boat to Point 1", "Boat to Point 2", "Boat to Point 3", "Boat to Point 4", "Local to Point 3", "Local to Point 2", "Local to Point 1", "Local to Point 0", "Local to Point 4": Value Change {
        # "save the current GPS location to one of the saved points."
        n76 = event-data() -> ()  [unwired: 1 in, 1 out]
        n77 = Build Array("Boat to Point 0", "Boat to Point 1", "Boat to Point 2", "Boat to Point 3", "Boat to Point 4") -> (w213:bool[])
        n78 = Build Array("Local to Point 0", "Local to Point 1", "Local to Point 2", "Local to Point 3", "Local to Point 4") -> (w204:bool[])
        n79 = for {
          tunnel: w213 -> [w226] mode=indexing
          i -> [w225]
          n80 = case shown="True" w226 {
            tunnel: w225 -> [_ w228]
            frame False {
            }
            frame True {
              # "load from boat GPS"
              n81 = local read "Stored Locations Array"() -> (w230:T5[])
              n82 = local read "Robot UTM Location"() -> (w227:T5)
              n83 = Replace Array Subset(array=w230, new element=w227, index=w228) -> (w229:T5[])
              n84 = local write "Stored Locations Array"(w229) -> ()
            }
          }
        }
        n85 = for {
          tunnel: w204 -> [w220] mode=indexing
          i -> [w219]
          n86 = case shown="True" w220 {
            tunnel: w219 -> [_ w221]
            frame False {
            }
            frame True {
              # "load from local GPS"
              n87 = local read "Stored Locations Array"() -> (w223:T5[])
              n88 = global read "2 Global.vi" "Robot UTM Location"() -> (w222:T5)
              n89 = Replace Array Subset(array=w223, new element=w222, index=w221) -> (w224:T5[])
              n90 = local write "Stored Locations Array"(w224) -> ()
            }
          }
        }
      }
      event "Update Constants": Value Change {
        # "To add a set of tuning constants, add a control constant in the cluster constant\nadd the control to the front panel and wire it into the bundler in the true case here; the  0x2 command\nreceive block will need to be edited as well as the TuningConstants global"
        n91 = event-data() -> ()  [unwired: 1 in, 1 out]
        n92 = case shown="True" "Update Constants" {
          tunnel: w234 -> [w238 w244]
          tunnel: w233 -> [w237 w243]
          tunnel: [w238 w242] -> w232
          tunnel: [w237 w241] -> w231
          frame False {
          }
          frame True {
            n93 = Bundle By Name(cluster=T45 {"OCU Command"=enum."Edit Control Values", "Data"=variant}, "Data"="Tuning Values") -> (w240:T45)
            n94 = call "Write.vi"("error in (no error)"=w243, "element"=w240, "NetworkStreamWriter in"=w244) -> ("error out"=w241:errorcluster, "NetworkStreamWriter out"=w242:refnum<class "NetworkStreamWriter.lvclass">)  [unwired: 7 in]
          }
        }
      }
      event "Log message": Key Up {
        # "Remove carriage\nreturn."
        # "Enter key?"
        n95 = event-data() -> ("ScanCode"=w247:i16)  [unwired: 1 in, 2 out]
        n96 = Equal?(x=w247, y=i16 28) -> (x = y?=w256:bool)
        n97 = Search and Replace String(replace all?=TRUE ("replace all? (F)"), input string="Log message", search string="\n" ("string"), replace string="") -> (result string=w253:string)  [unwired: 4 in, 3 out]
        n98 = case "Was the log message entered?" shown="True" w256 {
          tunnel: [w260 w269] -> w251
          tunnel: [w259 w268] -> w248
          tunnel: w250 -> [w259 w263]
          tunnel: w249 -> [w260 w267]
          tunnel: w253 -> [_ w264]
          frame False {
          }
          frame True {
            n99 = To Variant(anything=w264) -> (Variant=w271:variant)
            n100 = property on="Log message" class="Str"(error in=w263, "Value"="") -> (error out=w262:errorcluster)  [unwired: 1 in, 1 out]
            n101 = Bundle By Name(cluster=T45 {"OCU Command"=enum."Log Message", "Data"=variant}, "Data"=w271) -> (w270:T45)
            n102 = To Variant(anything=w270) -> (Variant=w265:variant)
            n103 = call "Write.vi"("error in (no error)"=w262, "element"=w265, "NetworkStreamWriter in"=w267) -> ("error out"=w268:errorcluster, "NetworkStreamWriter out"=w269:refnum<class "NetworkStreamWriter.lvclass">)  [unwired: 7 in]
          }
        }
      }
      event "Save Waypoints\nand PoI": Value Change {
        n104 = event-data() -> ()  [unwired: 1 in, 1 out]
        n105 = case "Save MDF" shown="True" "Save Waypoints\nand PoI" {
          frame False {
          }
          frame True {
            n106 = local read "Global No Sail Circles"() -> (w276:T34[])
            n107 = local read "Mission Object Array"() -> (w277:refnum<class "GenericMission.lvclass">[])
            n108 = call "0-Write MDF.vi"("Global No Sail Circles"=w276, "Missions (Object Array)"=w277) -> ()  [unwired: 3 in, 1 out]
          }
        }
      }
      event "Load MDF": Value Change {
        n109 = event-data() -> ()  [unwired: 1 in, 1 out]
        n110 = case "Load MDF" shown="True" "Load MDF" {
          tunnel: w281 -> [w284 w287]
          tunnel: [w284 w294] -> w280
          tunnel: w279 -> [w285 w289]
          tunnel: [w285 w292] -> w278
          frame False {
          }
          frame True {
            w291 = T45 {"OCU Command"=enum."Reset Missions/Waypts", "Data"=variant}  # clear missions
            n111 = To Variant(anything=w291) -> (Variant=w290:variant)
            n112 = call "Write.vi"("error in (no error)"=w287, "element"=w290, "NetworkStreamWriter in"=w289) -> ("error out"=w286:errorcluster, "NetworkStreamWriter out"=w288:refnum<class "NetworkStreamWriter.lvclass">)  [unwired: 7 in]
            n113 = call "0-Read MDF.vi"("Error in"=w286, "MDF file path"="Mission Def Filepath") -> ("Error out"=w296:errorcluster, "Global No Sail Circles"=w298:T34[], "Missions (Object Array)"=w297:refnum<class "GenericMission.lvclass">[])  [unwired: 1 in]
            n114 = for {
              tunnel: w297 -> [w309] mode=indexing
              shift-right: [w315] -> w295
              shift-left: w296 -> [w311]
              shift-right: [w313] -> w293
              shift-left: w288 -> [w314]
              n115 = Flatten To String(anything=w309, error in (no error)=w311) -> (data string=w310:string, error out=w312:errorcluster)  [unwired: 2 in, 1 out]
              n116 = To Variant(anything=w310) -> (Variant=w317:variant)
              n117 = Bundle By Name(cluster=T45 {"OCU Command"=enum."Add Mission", "Data"=variant}, "Data"=w317) -> (w318:T45)
              n118 = To Variant(anything=w318) -> (Variant=w316:variant)
              n119 = call "Write.vi"("error in (no error)"=w312, "element"=w316, "NetworkStreamWriter in"=w314) -> ("error out"=w315:errorcluster, "NetworkStreamWriter out"=w313:refnum<class "NetworkStreamWriter.lvclass">)  [unwired: 7 in]
            }
            n120 = local write "Mission Object Array"(w297) -> ()
            n121 = local write "Global No Sail Circles"(w298) -> ()
            n122 = for {
              tunnel: w298 -> [w301] mode=indexing
              shift-right: [w304] -> w294
              shift-left: w295 -> [w300]
              shift-right: [w302] -> w292
              shift-left: w293 -> [w303]
              n123 = To Variant(anything=w301) -> (Variant=w306:variant)
              n124 = Bundle By Name(cluster=T45 {"OCU Command"=enum."Add Global No-Sail", "Data"=variant}, "Data"=w306) -> (w307:T45)
              n125 = To Variant(anything=w307) -> (Variant=w305:variant)
              n126 = call "Write.vi"("error in (no error)"=w300, "element"=w305, "NetworkStreamWriter in"=w303) -> ("error out"=w304:errorcluster, "NetworkStreamWriter out"=w302:refnum<class "NetworkStreamWriter.lvclass">)  [unwired: 7 in]
            }
          }
        }
      }
      event "Reset Missions/Waypts": Value Change {
        n127 = event-data() -> ()  [unwired: 1 in, 1 out]
        n128 = case "Reset Missions" shown="True" "Reset Missions/Waypts" {
          tunnel: w323 -> [w327 w333]
          tunnel: w322 -> [w326 w332]
          tunnel: [w327 w331] -> w321
          tunnel: [w326 w330] -> w320
          frame False {
          }
          frame True {
            n129 = To Variant(anything=T45 {"OCU Command"=enum."Reset Missions/Waypts", "Data"=variant}) -> (Variant=w328:variant)
            n130 = call "Write.vi"("error in (no error)"=w332, "element"=w328, "NetworkStreamWriter in"=w333) -> ("error out"=w330:errorcluster, "NetworkStreamWriter out"=w331:refnum<class "NetworkStreamWriter.lvclass">)  [unwired: 7 in]
          }
        }
      }
      event Value Change {
        # "gray out the appropriate numeric controls"
        # "set input tool"
        # "Adjust OCU controls for the correct mission input style"
        n131 = event-data() -> ("NewVal"=w339:T15)  [unwired: 1 in]
        n132 = case shown="\"Station Keeping\"" w339 {
          tunnel: [T47."Enabled" ("Disabled") w343 T47."Enabled" ("Disabled")] -> w338
          tunnel: [T47."Disabled and Grayed Out" ("Disabled") w343 T47."Enabled" ("Disabled")] -> w337
          frame "Go to Waypoint", Default {
          }
          frame "Pass Between Buoys", "Global No-Sail Zone" {
            w343 = T47."Disabled and Grayed Out" ("Disabled")
            # "\"Pass Between Buoys\"\nhas neither input"
          }
          frame "Station Keeping" {
          }
        }
        n133 = case shown="\"Pass Between Buoys\", \"Global No-Sail Zone\"" w339 {
          tunnel: [w346 w347 w348] -> w340
          frame "Go to Waypoint", Default {
            w346 = u32 1 items=["Zoom Tool"=8, "Selection Tool"=0, "Pan Tool"=9, "Point Tool"=1, "Line Tool"=2, "Rectangle Tool"=3, "Rotated Rectangle Tool"=12, "Polyline Tool"=10, "Polygon Tool"=5, "Freehand Tool"=11, "Closed Freehand Tool"=6, "Ellipse Tool"=4, "Annulus Tool"=7] ("Current ROI Tool")
          }
          frame "Station Keeping" {
            w347 = u32 2 items=["Zoom Tool"=8, "Selection Tool"=0, "Pan Tool"=9, "Point Tool"=1, "Line Tool"=2, "Rectangle Tool"=3, "Rotated Rectangle Tool"=12, "Polyline Tool"=10, "Polygon Tool"=5, "Freehand Tool"=11, "Closed Freehand Tool"=6, "Ellipse Tool"=4, "Annulus Tool"=7] ("Current ROI Tool")
          }
          frame "Pass Between Buoys", "Global No-Sail Zone" {
            w348 = u32 2 items=["Zoom Tool"=8, "Selection Tool"=0, "Pan Tool"=9, "Point Tool"=1, "Line Tool"=2, "Rectangle Tool"=3, "Rotated Rectangle Tool"=12, "Polyline Tool"=10, "Polygon Tool"=5, "Freehand Tool"=11, "Closed Freehand Tool"=6, "Ellipse Tool"=4, "Annulus Tool"=7] ("Current ROI Tool")
          }
        }
        n134 = property on="Tolerance" class="DigNum (strict)"("DisabledEnum"=w338) -> ()  [unwired: 2 in, 2 out]
        n135 = property on="Time(s)" class="DigNum (strict)"("DisabledEnum"=w337) -> ()  [unwired: 2 in, 2 out]
        n136 = property on="Mission Map" class="ImageControl"("Current ROI Tool"=w340) -> ()  [unwired: 2 in, 2 out]
      }
      event "Mission Map": Mouse Up {
        # "add a waypoint to the list"
        n137 = event-data() -> ()  [unwired: 1 in, 1 out]
        n138 = global read "OCUtoSim.vi" "Pause Simulator?"() -> (w349:bool)
        n139 = case shown="True" w349 {
          tunnel: w357 -> [w366 w489]
          tunnel: w356 -> [w365 w487]
          tunnel: [w364 w488] -> w355
          tunnel: [w363 w490] -> w354
          tunnel: w353 -> [w362 w490]
          tunnel: w352 -> [w361 _]
          tunnel: w351 -> [w360 _]
          tunnel: w350 -> [w359 _]
          frame False {
            n140 = case shown="\"Go to Waypoint\", Default" w361 {
              selector: w361 -> [_ _ w440 _ _]
              tunnel: w366 -> [w376 w402 w447 w465 w485]
              tunnel: [w374 w412 w444 w456 w476] -> w364
              tunnel: w365 -> [w375 w399 w429 w451 w483]
              tunnel: w360 -> [w369 _ w441 _ w466]
              tunnel: [w372 w410 w433 w459 w477] -> w363
              tunnel: w362 -> [w371 w409 w430 w460 w475]
              tunnel: w359 -> [_ _ _ _ w467]
              frame "Go to Waypoint", Default {
                n141 = property on="Mission Map" class="ImageControl"(error in=w376) -> (error out=w378:errorcluster, "Last Mouse Position"=w377:cluster{"X":i32, "Y":i32})  [unwired: 1 in, 1 out]
                n142 = call "Helper - Image To UTM.vi"("Image Descriptor"=w375, "Pixel Coordinates"=w377) -> ("UTM Location"=w367:T5)  [unwired: 1 in, 1 out]
                n143 = invoke on="Mission Map" class="ImageControl" method="Clear ROI"(error in=w378) -> (error out=w373:errorcluster)  [unwired: 2 in, 2 out]
                n144 = disable-structure shown="Enabled" {
                  disable-tunnel: w369 -> [w385 w388]
                  disable-tunnel: [w381 w392] -> w368
                  disable-tunnel: w367 -> [w379 w387]
                  frame Enabled {
                    n145 = call "Initialize.vi"("Tolerance (m)"=w385, "Drive Location"=w379) -> ("Drive out"=w380:refnum<class "DriveTo.lvclass">)  [unwired: 8 in, 1 out]
                    n146 = Flatten To String(anything=w380) -> (data string=w382:string)  [unwired: 3 in, 2 out]
                    n147 = To Variant(anything=w382) -> (Variant=w383:variant)
                    n148 = Bundle By Name(cluster=T45 {"OCU Command"=enum."Add Mission", "Data"=variant}, "Data"=w383) -> (w381:T45)
                  }
                  frame Disabled {
                    n149 = call "init_waypoint.vi"("Coords"=w387, "Tolerance (m)"=w388) -> ("Waypoint Out"=w386:refnum<class "Waypoint.lvclass">)  [unwired: 9 in]
                    n150 = Flatten To String(anything=w386) -> (data string=w389:string)  [unwired: 3 in, 2 out]
                    n151 = To Variant(anything=w389) -> (Variant=w390:variant)
                    n152 = Bundle By Name(cluster=T45 {"OCU Command"=enum."Set waypoint number", "Data"=variant}, "Data"=w390) -> (w392:T45)
                  }
                }
                n153 = To Variant(anything=w368) -> (Variant=w370:variant)
                n154 = call "Write.vi"("error in (no error)"=w373, "element"=w370, "NetworkStreamWriter in"=w371) -> ("error out"=w374:errorcluster, "NetworkStreamWriter out"=w372:refnum<class "NetworkStreamWriter.lvclass">)  [unwired: 7 in]
              }
              frame "Global No-Sail Zone" {
                n155 = property on="Mission Map" class="ImageControl"(error in=w402) -> (error out=w401:errorcluster, "ROI"=w403:T49)  [unwired: 1 in, 1 out]
                n156 = call "helper- line ROI to 2 UTM Pts.vi"("ROI"=w403, "Image Descriptor"=w399) -> ("Endpoint UTM 2"=w398:T5, "Endpoint UTM 1"=w400:T5)
                n157 = Unbundle By Name(w398) -> ("East"=w396:dbl, "North"=w397:dbl)
                n158 = Unbundle By Name(w400) -> ("UTM Zone"=w404:dbl, "Hemisphere"=w405:enum16{"North", "South"}, "East"=w394:dbl, "North"=w395:dbl)
                n159 = call "2 XYPointsToDistanceAndAngle.vi"("East 2"=w397, "North 2"=w396, "East 1"=w395, "North 1"=w394) -> ("Distance"=w393:dbl)  [unwired: 6 in, 1 out]
                n160 = invoke on="Mission Map" class="ImageControl" method="Clear ROI"(error in=w401) -> (error out=w411:errorcluster)  [unwired: 2 in, 2 out]
                n161 = disable-structure shown="Enabled" {
                  disable-tunnel: w393 -> [w418 w424]
                  disable-tunnel: [w420 w428] -> w407
                  disable-tunnel: T34 {"UTM Zone"=0.0, "Hemisphere"=enum."North", "East"=0.0, "North"=0.0, "Radius"=0.0} ("UTM Location") -> [w419 _]
                  disable-tunnel: w395 -> [w417 _]
                  disable-tunnel: w394 -> [w416 _]
                  disable-tunnel: w405 -> [w415 _]
                  disable-tunnel: w404 -> [w414 _]
                  frame Enabled {
                    n162 = Bundle By Name(cluster=w419, "UTM Zone"=w414, "Hemisphere"=w415, "East"=w416, "North"=w417, "Radius"=w418) -> (w413:T34)
                    n163 = To Variant(anything=w413) -> (Variant=w421:variant)
                    n164 = Bundle By Name(cluster=T45 {"OCU Command"=enum."Add Global No-Sail", "Data"=variant}, "Data"=w421) -> (w420:T45)
                  }
                  frame Disabled {
                    n165 = call "init_waypoint.vi"("Tolerance (m)"=w424) -> ("Waypoint Out"=w423:refnum<class "Waypoint.lvclass">)  [unwired: 10 in]
                    n166 = Flatten To String(anything=w423) -> (data string=w425:string)  [unwired: 3 in, 2 out]
                    n167 = To Variant(anything=w425) -> (Variant=w426:variant)
                    n168 = Bundle By Name(cluster=T45 {"OCU Command"=enum."Set waypoint number", "Data"=variant}, "Data"=w426) -> (w428:T45)
                  }
                }
                n169 = To Variant(anything=w407) -> (Variant=w408:variant)
                n170 = call "Write.vi"("error in (no error)"=w411, "element"=w408, "NetworkStreamWriter in"=w409) -> ("error out"=w412:errorcluster, "NetworkStreamWriter out"=w410:refnum<class "NetworkStreamWriter.lvclass">)  [unwired: 7 in]
              }
              frame "Round Buoy Starboard", "Round Buoy Port" {
                n171 = property on="Mission Map" class="ImageControl"(error in=w447) -> (error out=w449:errorcluster, "Last Mouse Position"=w448:cluster{"X":i32, "Y":i32})  [unwired: 1 in, 1 out]
                n172 = Equal?(x=w440, y=Mission_Type_Radio_Buttons."Round Buoy Port" ("Mission Type 2")) -> (x = y?=w435:bool)
                n173 = call "Helper - Image To UTM.vi"("Image Descriptor"=w429, "Pixel Coordinates"=w448) -> ("UTM Location"=w442:T5)  [unwired: 1 in, 1 out]
                n174 = invoke on="Mission Map" class="ImageControl" method="Clear ROI"(error in=w449) -> (error out=w444:errorcluster)  [unwired: 2 in, 2 out]
                n175 = Select(t=enum16{"Starboard", "Port"}."Port" ("Round side?"), s=w435, f=enum16{"Starboard", "Port"}."Starboard" ("Round side?")) -> (s? t:f=w436:enum16{"Starboard", "Port"})
                n176 = call "Initialize.vi"("Tolerance (m)"=w441, "Round side?"=w436, "Buoy to Round"=w442) -> ("RoundBuoys out"=w434:refnum<class "RoundBuoy.lvclass">)  [unwired: 7 in, 1 out]
                n177 = Flatten To String(anything=w434) -> (data string=w443:string)  [unwired: 3 in, 2 out]
                n178 = To Variant(anything=w443) -> (Variant=w445:variant)
                n179 = Bundle By Name(cluster=T45 {"OCU Command"=enum."Add Mission", "Data"=variant}, "Data"=w445) -> (w431:T45)
                n180 = To Variant(anything=w431) -> (Variant=w432:variant)
                n181 = call "Write.vi"("element"=w432, "NetworkStreamWriter in"=w430) -> ("NetworkStreamWriter out"=w433:refnum<class "NetworkStreamWriter.lvclass">)  [unwired: 8 in, 1 out]
              }
              frame "Pass Between Buoys" {
                # "build Pass Between Buoys mission"
                n182 = property on="Mission Map" class="ImageControl"(error in=w465) -> (error out=w457:errorcluster, "ROI"=w450:T49)  [unwired: 1 in, 1 out]
                n183 = invoke on="Mission Map" class="ImageControl" method="Clear ROI"(error in=w457) -> (error out=w458:errorcluster)  [unwired: 2 in, 2 out]
                n184 = call "helper- line ROI to 2 UTM Pts.vi"("ROI"=w450, "Image Descriptor"=w451) -> ("Endpoint UTM 2"=w453:T5, "Endpoint UTM 1"=w452:T5)
                n185 = call "Initialize.vi"("Buoy Pass 2"=w453, "Buoy Pass 1"=w452) -> ("PassBuoys out"=w454:refnum<class "PassBuoys.lvclass">)  [unwired: 8 in, 1 out]
                n186 = Flatten To String(anything=w454) -> (data string=w462:string)  [unwired: 3 in, 2 out]
                n187 = To Variant(anything=w462) -> (Variant=w463:variant)
                n188 = Bundle By Name(cluster=T45 {"OCU Command"=enum."Add Mission", "Data"=variant}, "Data"=w463) -> (w461:T45)
                n189 = To Variant(anything=w461) -> (Variant=w455:variant)
                n190 = call "Write.vi"("error in (no error)"=w458, "element"=w455, "NetworkStreamWriter in"=w460) -> ("error out"=w456:errorcluster, "NetworkStreamWriter out"=w459:refnum<class "NetworkStreamWriter.lvclass">)  [unwired: 7 in]
              }
              frame "Station Keeping" {
                # "user inputs two points as a line and we convert it to a square"
                n191 = property on="Mission Map" class="ImageControl"(error in=w485) -> (error out=w473:errorcluster, "ROI"=w484:T49)  [unwired: 1 in, 1 out]
                n192 = call "helper- line ROI to 2 UTM Pts.vi"("ROI"=w484, "Image Descriptor"=w483) -> ("Endpoint UTM 2"=w468:T5, "Endpoint UTM 1"=w469:T5)
                n193 = call "helper - UTM line to Square.vi"("Endpoint 2, UTM"=w468, "Endpoint 1, UTM"=w469) -> ("Endpoint 4, UTM"=w471:T5, "Endpoint 3, UTM"=w470:T5)
                n194 = invoke on="Mission Map" class="ImageControl" method="Clear ROI"(error in=w473) -> (error out=w474:errorcluster)  [unwired: 2 in, 2 out]
                n195 = call "Initialize.vi"("Tolerance (m)"=w466, "Duration (s)"=w467, "Buoy SE"=w468, "Buoy SW"=w469, "Buoy NE"=w471, "Buoy NW"=w470) -> ("StationKeeping out"=w472:refnum<class "StationKeeping.lvclass">)  [unwired: 4 in, 1 out]
                n196 = Flatten To String(anything=w472) -> (data string=w480:string)  [unwired: 3 in, 2 out]
                n197 = To Variant(anything=w480) -> (Variant=w481:variant)
                n198 = Bundle By Name(cluster=T45 {"OCU Command"=enum."Add Mission", "Data"=variant}, "Data"=w481) -> (w479:T45)
                n199 = To Variant(anything=w479) -> (Variant=w478:variant)
                n200 = call "Write.vi"("error in (no error)"=w474, "element"=w478, "NetworkStreamWriter in"=w475) -> ("error out"=w476:errorcluster, "NetworkStreamWriter out"=w477:refnum<class "NetworkStreamWriter.lvclass">)  [unwired: 7 in]
              }
            }
          }
          frame True {
            # "While we're paused, if you click on the map, that sets the new location and flushes velocity/rate of turn"
            n201 = global read "OCUtoSim.vi" "Move boat?"() -> (w486:bool)
            n202 = case shown="True" w486 {
              tunnel: w489 -> [w491 w498]
              tunnel: [w491 w497] -> w488
              tunnel: w487 -> [_ w494]
              frame False {
              }
              frame True {
                n203 = property on="Mission Map" class="ImageControl"(error in=w498) -> (error out=w499:errorcluster, "Last Mouse Position"=w496:cluster{"X":i32, "Y":i32})  [unwired: 1 in, 1 out]
                n204 = invoke on="Mission Map" class="ImageControl" method="Clear ROI"(error in=w499) -> (error out=w497:errorcluster)  [unwired: 2 in, 2 out]
                n205 = call "Helper - Image To UTM.vi"("Image Descriptor"=w494, "Pixel Coordinates"=w496) -> ("UTM Location"=w495:T5)  [unwired: 1 in, 1 out]
                n206 = global write "2 Global.vi" "Robot\nRate of Turn"(T21 0.0 ("Robot\nRate of Turn")) -> ()
                n207 = global write "2 Global.vi" "Robot UTM Location"(w495) -> ()
                n208 = global write "2 Global.vi" "Robot Velocity"(T20 {"East"=0.0, "North"=0.0} ("Robot Velocity")) -> ()
              }
            }
          }
        }
      }
      event "Pause Simulator?": Value Change {
        # "Why are there so many controls......."
        # "I'm leaving the tuning constants\nas is because they'll change anyway."
        # "Disable controls when paused because it doesn't make sense to change them while paused!"
        n209 = event-data() -> ("NewVal"=w501:bool)  [unwired: 1 in, 1 out]
        n210 = case shown="True" w500 {
          tunnel: w501 -> [_ w505]
          frame False {
          }
          frame True {
            n211 = global write "OCUtoSim.vi" "Pause Simulator?"(w505) -> ()
            n212 = Select(t=T47."Disabled and Grayed Out" ("Disabled"), s=w505, f=T47."Enabled" ("Disabled")) -> (s? t:f=w506:T47)
            n213 = property on="OVERRIDE RUDDER?" class="Bool (strict)"("DisabledEnum"=w506) -> ()  [unwired: 2 in, 2 out]
            n214 = property on="OVERRIDE SAIL?" class="Bool (strict)"("DisabledEnum"=w506) -> ()  [unwired: 2 in, 2 out]
            n215 = property on="Load MDF" class="Bool"("DisabledEnum"=w506) -> ()  [unwired: 2 in, 2 out]
            n216 = property on="Location of THINK" class="CmbBox (strict)"("DisabledEnum"=w506) -> ()  [unwired: 2 in, 2 out]
            n217 = property on="Map Name" class="CmbBox (strict)"("DisabledEnum"=w506) -> ()  [unwired: 2 in, 2 out]
            n218 = property on="Mission Def Filepath" class="Path"("DisabledEnum"=w506) -> ()  [unwired: 2 in, 2 out]
            n219 = property on="Setpoints to boat" class="Clust (strict)"("DisabledEnum"=w506) -> ()  [unwired: 2 in, 2 out]
            n220 = property on="Mission Entry Type" class="RadioBtnsControl (strict)"("DisabledEnum"=w506) -> ()  [unwired: 2 in, 2 out]
          }
        }
      }
      event "Set Wind Speed": Value Change {
        # "Control the wind speed for the simulator from the OCU.\nTechnically pause simulator should never be true when it's not the simulator.\nBut do you really want to risk it?"
        n221 = event-data() -> ("NewVal"=w516:dbl)  [unwired: 1 in, 1 out]
        n222 = global read "OCUtoSim.vi" "Pause Simulator?"() -> (w513:bool)
        n223 = Not(x=w513) -> (.not. x?=w512:bool)
        n224 = And(x=w514, y=w512) -> (x .and. y?=w515:bool)
        n225 = case shown="True" w515 {
          tunnel: w516 -> [_ w517]
          frame False {
          }
          frame True {
            n226 = global write "2 Global.vi" "Absolute Wind\nSpeed"(w517) -> ()
          }
        }
      }
      event "Set Wind Direction": Value Change {
        # "If we're on the simulator AND it isn't paused, let us change\nthe wind direction."
        n227 = event-data() -> ("NewVal"=w521:dbl)  [unwired: 1 in, 1 out]
        n228 = global read "OCUtoSim.vi" "Pause Simulator?"() -> (w523:bool)
        n229 = Not(x=w523) -> (.not. x?=w525:bool)
        n230 = And(x=w524, y=w525) -> (x .and. y?=w522:bool)
        n231 = case shown="True" w522 {
          tunnel: w521 -> [_ w526]
          frame False {
          }
          frame True {
            n232 = global write "2 Global.vi" "Absolute Wind\nDirection (º)"(w526) -> ()
          }
        }
      }
      event "Set Water Current Speed", "Set Water Current Direction": Value Change {
        # "set the water current based on the controls. Angles correspond to how they look on the dial."
        n233 = event-data() -> ()  [unwired: 1 in, 1 out]
        n234 = case "Only allow water current to be set in simulation." shown="True" w527 {
          frame False {
          }
          frame True {
            n235 = global read "2 Global.vi" "Absolute Water Current Vector"() -> (w538:T23)
            n236 = expression code="(x/180.0)*pi" "degrees to radians"("Set Water Current Direction") -> (w536:dbl)
            n237 = Cosine(x=w536) -> (cos(x)=w534:dbl)
            n238 = Sine(x=w536) -> (sin(x)=w535:dbl)
            n239 = Multiply(x="Set Water Current Speed", y=w534) -> (x*y=w531:dbl)
            n240 = Multiply(x=w535, y="Set Water Current Speed") -> (x*y=w532:dbl)
            n241 = Bundle By Name(cluster=w538, "North"=w532, "East"=w531) -> (w539:T23)
            n242 = global write "2 Global.vi" "Absolute Water Current Vector"(w539) -> ()
          }
        }
      }
      event "Move boat?": Value Change {
        # "If we're on the simulator, and we're pausing the simulator, and we want to move the boat, let us move the boat."
        n243 = event-data() -> ("NewVal"=w546:bool)  [unwired: 1 in, 1 out]
        n244 = global read "OCUtoSim.vi" "Pause Simulator?"() -> (w543:bool)
        n245 = Compound Arithmetic op=AND(w546, w543, w544) -> (w545:bool)
        n246 = global write "OCUtoSim.vi" "Move boat?"(w545) -> ()
      }
      event "Set Boat Heading": Value Change {
        n247 = event-data() -> ("NewVal"=w550:dbl)  [unwired: 1 in, 1 out]
        n248 = global read "OCUtoSim.vi" "Move boat?"() -> (w553:bool)
        n249 = global read "OCUtoSim.vi" "Pause Simulator?"() -> (w552:bool)
        n250 = Compound Arithmetic op=AND(w554, w553, w552) -> (w551:bool)
        n251 = case shown="True" w551 {
          tunnel: w550 -> [_ w555]
          frame False {
          }
          frame True {
            n252 = global write "2 Global.vi" "Robot\nHeading"(w555) -> ()
          }
        }
      }
    }
    n253 = local read "Setpoints to boat"() -> (w44:T27)
    n254 = local read "OVERRIDE RUDDER?"() -> (w50:bool)
    n255 = local read "OVERRIDE SAIL?"() -> (w45:bool)
    n256 = Unbundle By Name(w52) -> ("Sail Position"=w47:T28, "Rudder Angle"=w48:T29)
    n257 = Unbundle By Name(w44) -> ("Sail Position"=w43:T28, "Rudder Angle"=w42:T29)
    n258 = call "eStopShared.vi"("Command"=eStopCommand."Set E-Stop", "E-Stop"="Stop") -> ("E-Stop Out"=w57:bool)  [unwired: 8 in, 1 out]
    n259 = Select(t=w47, s=w45, f=w43) -> (s? t:f=→"Sail Position":T28)
    n260 = Select(t=w48, s=w50, f=w42) -> (s? t:f=→"Rudder Position":T29)
  }
  n261 = while "Read from network stream to update" {
    shift-right: [w611] -> w29
    shift-left: w32 -> [w606]
    shift-right: [w604] -> w28
    shift-left: w6 -> [w605]
    tunnel: w27 -> [w608]
    tunnel: w14 -> [w607]
    stop <- w609 stop-if-true
    n262 = call "IsConnected.vi"("error in (no error)"=w605, "NetworkStreamReader in"=w606) -> ("error out"=w600:errorcluster, "Connected?"=→"Connected?":bool, "NetworkStreamReader out"=w601:refnum<class "NetworkStreamReader.lvclass">)  [unwired: 7 in]
    n263 = call "Read.vi"("Read Type"=readType."Most current", "error in (no error)"=w600, "NetworkStreamReader in"=w601) -> ("error out"=w597:errorcluster, "element"=w596:variant, "NetworkStreamReader out"=w611:refnum<class "NetworkStreamReader.lvclass">)  [unwired: 4 in, 2 out]
    n264 = Variant To Data(error in=w597, type=T36 {"Sensor Status"={"Sensor Connected"=FALSE, "Sensor Initialized"=FALSE, "Sensor OK"=FALSE, "Latest Error String"="", "GPS Lock"=FALSE}, "Battery Voltage"=0.0, "Rudder Actuator Status"={"Actuator Connected"=FALSE}, "Sail Actuator Status"={"Actuator Connected"=FALSE}, "Which Boat Am I?"=enum."Axiom; Blackbody Radiation", "Robot Velocity"={"East"=0.0, "North"=0.0}, "Robot UTM Location"={"UTM Zone"=0.0, "Hemisphere"=enum."North", "East"=0.0, "North"=0.0}, "Robot\nHeading "=0.0, "Robot\nRate of Turn"=0.0, "Robot Pitch/Roll"={"Pitch"=0.0, "Roll"=0.0}, "Apparent Wind"={"Toward Fore"=0.0, "Toward Starboard"=0.0}, "Apparent Wind\nSpeed"=0.0, "Apparent Wind\nDirection (º)"=0.0, "Absolute Wind"={"East"=0.0, "North"=0.0}, "Absolute Wind\nDirection (º)"=0.0, "Absolute Wind\nSpeed"=0.0, "Absolute Water Current Vector"={"Direction"=0.0, "Magnitude"=0.0}, "Rudder Angle"=0.0, "Sail Position"=0.0, "Manual Override Cluster"={"Override Active Rudder"=FALSE, "Setpoints"={"Sail Position"=0.0, "Rudder Angle"=0.0}, "Override Active Sail"=FALSE}, "Setpoints to boat"={"Sail Position"=0.0, "Rudder Angle"=0.0}, "Current Waypoint"=0, "Think freq."=0.0, "Sense freq."=0.0, "Act freq."=0.0, "E-stop freq."=0.0, "Network \nfreq."=0.0, "Network \nLoop Iterations"=0, "E-Stop"=FALSE, "Serialized Waypoint Array"="", "Serialized Mission Queue Elements"="", "Goodness Functions"={0.0, 0.0, []}, "Global No Sail Circles"=[], "Optimal Heading"=0.0, "Crossing Wind"=FALSE, "Estimated Error"=0.0, "Don't Tip?"=FALSE, "Tacking Attempt"={"attempting tack"=FALSE, "tacking attempt\ntime remaining"=0.0}} ("RIO->OCU update data"), Variant=w596) -> (data=w594:T36, error out=w599:errorcluster)
    n265 = Unbundle By Name(w594) -> ("Estimated Error"=→"Estimated Error":dbl, "Sensor Status"=→"Wind Sensor Status":T1, "Battery Voltage"=→"Battery Voltage":dbl, "Which Boat Am I?"=→"Which Boat Am I?":T12, "Robot Velocity"=w562:T20, "Robot UTM Location"=w574:T5, "Robot\nHeading"=w570:T16, "Robot\nRate of Turn"=→"Robot\nRate of Turn":T21, "Robot Pitch/Roll"=→"Robot Pitch/Roll":T22, "Apparent Wind"=→"Apparent Wind":T26, "Apparent Wind\nSpeed"=→"Apparent Wind Speed":T25, "Apparent Wind\nDirection (º)"=→"Apparent Wind Direction" →"Apparent Wind Direction\nPoint of Sail":T24, "Absolute Wind"=→"Absolute Wind":T23, "Rudder Angle"=→"Rudder Angle":T29, "Sail Position"=w585:T28, "Manual Override Cluster"=→"Manual Override":T31, "Setpoints to boat"=→"Setpoints to boat":T27, "Serialized Mission Queue Elements"=w581:string, "Global No Sail Circles"=w578:T34[], "Optimal Heading"=w573:dbl, "Goodness Functions"=w577:T41, "Current Waypoint"=w564:T30, "Serialized Waypoint Array"=w584:string, "Crossing Wind"=→"Crossing Wind":bool, "Don't Tip?"=→"Don't Tip?":bool)  [unwired: 7 out]
    "Robot UTM Location" <- w574
    "Robot Heading" <- w570
    "Robot Velocity" <- w562
    "Sail Position" <- w585
    "Current Waypoint" <- w564
    "Global No Sail Circles" <- w578
    "Heading" <- w570
    n266 = Bundle("Image Ref Out"=w608, "Image Descriptor"=w607) -> (w572:T51)  [unwired: 1 in]
    n267 = call "Deserialize Waypoint Array.vi"("Serialized Waypoint Array"=w584) -> ("Waypoints Object Array"=w582:T33, "Waypoints Array"=→"Waypoints Array":T32[])  [unwired: 9 in]
    "Waypoints Object Array" <- w582
    n268 = call "deserializeMissionArray.vi"("Serialized Mission Array"=w581) -> ("Mission Object Array"=w565:refnum<class "GenericMission.lvclass">[])  [unwired: 9 in, 1 out]
    "Mission Object Array" <- w565
    n269 = call "Velocity Converter- dx-dy to magnitude-heading.vi"("Vector In"=w562) -> ("Magnitude Out"=→"Robot Speed (m/s)":dbl)  [unwired: 9 in, 1 out]
    n270 = call "0-Do Overlays.vi"("Image Reference\nand Descriptor"=w572, "Missions"=w565, "No Sail Circles"=w578, "Waypoints"=w582, "Current Waypoint #"=w564, "Heading"=w570, "Sail Position"=w585, "Robot UTM Location"=w574, "Optimal Heading"=w573, "Font Size"="Overlay Font Size") -> ("Image out"=→"Mission Map":T11)  [unwired: 5 in]
    n271 = Array Size(array=w582) -> (size(s)=→"# of Waypts":i32)
    n272 = call "Helper - goodness polar plot.vi"("Plot Colors"="Plot Colors", "Goodness Fns In"=w577) -> ("Goodness Functions Polar Plot"=→"Goodness Functions":picture)  [unwired: 9 in]
    n273 = Index Array(array=w565, index=0) -> (element=w566:refnum<class "GenericMission.lvclass">)
    n274 = call-dynamic "getStatus.vi"("GenericMission in"=w566) -> ("Status"=→"Mission Status":string)  [unwired: 8 in, 2 out]
    n275 = Wait (ms)(milliseconds to wait=u32 50 ("millisecond multiple")) -> ()  [unwired: 1 out]
    n276 = call "eStopShared.vi"("Command"=eStopCommand."Get E-Stop", "Error In"=w599) -> ("Error Out"=w604:errorcluster, "E-Stop Out"=w609:bool)  [unwired: 8 in]
  }
  n277 = while {
    stop <- w621 stop-if-true
    n278 = global read "2 Global.vi" "Sensor Status"() -> (w619:T1)
    "Sensor Status" <- w619
    n279 = Unbundle By Name(w619) -> ("Sensor OK"=w615:T2, "Sensor Initialized"=w614:T2, "GPS Lock"=w612:T2)
    n280 = And(x=w615, y=w614) -> (x .and. y?=w613:T2)
    n281 = case shown="False" "Enable \nLocal GPS" {
      tunnel: w613 -> [_ w624]
      frame False {
        n282 = Wait Until Next ms Multiple(millisecond multiple=u32 100) -> ()  [unwired: 1 out]
      }
      frame True {
        n283 = case shown="False" w624 {
          tunnel: [w631 w633] -> w628
          tunnel: "GPS COM port" -> [w632 w633]
          tunnel: [w630 _] -> w626
          frame False {
            n284 = call "1A Helper - Init Sensor.vi"("VISA Refnum in"=w632) -> ("error out"=w630:errorcluster, "VISA Refnum out"=w631:refnum<visa-resource-name>)  [unwired: 8 in, 1 out]
          }
          frame True {
          }
        }
        n285 = call "1A Read Sensor Data.vi"("error (in)"=w626, "VISA resource name (in)"=w628) -> ("error (out)"=w625:errorcluster)  [unwired: 8 in, 1 out]
        n286 = case shown="Error" w625 {
          frame No Error {
          }
          frame Error {
            n287 = local write "Enable \nLocal GPS"(FALSE ("Enable \nLocal GPS")) -> ()
          }
        }
      }
    }
    n288 = call "eStopShared.vi"("Command"=eStopCommand."Get E-Stop") -> ("E-Stop Out"=w621:bool)  [unwired: 9 in, 1 out]
    n289 = Select(t=T47."Enabled" ("Disabled"), s=w612, f=T47."Disabled and Grayed Out" ("Disabled")) -> (s? t:f=w616:T47)
    n290 = property on="Local to Point 0" class="Bool"("DisabledEnum"=w616) -> ()  [unwired: 2 in, 2 out]
    n291 = property on="Local to Point 1" class="Bool"("DisabledEnum"=w616) -> ()  [unwired: 2 in, 2 out]
    n292 = property on="Local to Point 2" class="Bool"("DisabledEnum"=w616) -> ()  [unwired: 2 in, 2 out]
    n293 = property on="Local to Point 3" class="Bool"("DisabledEnum"=w616) -> ()  [unwired: 2 in, 2 out]
    n294 = property on="Local to Point 4" class="Bool"("DisabledEnum"=w616) -> ()  [unwired: 2 in, 2 out]
  }
  n295 = call "Close.vi"("error in (no error)"=w28, "NetworkStreamReader in"=w29) -> ()  [unwired: 9 in, 1 out]
  n296 = call "Close.vi"("error in (no error)"=w23, "NetworkStreamWriter in"=w24) -> ()  [unwired: 9 in, 1 out]
